vi "HighThroughputReactorCode.vi"() -> ()   [LabVIEW 2021]
uses:
  <vilib>/Utility/error.llb/DialogType.ctl
  839ea58d-a57c-48ce-b4c9-336fce4e4ed7.vi
panel:
  in  "Reactor Selector":T1(ring)
  in  "Stop Program":bool
  in  "Emergency Process Stop":bool
  in  "Reactor Tabs":T2(tab)
  in  "Time Elapsed (s) 1":dbl
  out "Current Cycle 1":string
  out "Completion 1":string
  out "Time Left 1":string="00:00:00"
  in  "Wait Before Start (s) 1":i32
  out "Pressure\nLimit\nTripped 1":bool
  out "Pressure\nTolerance\nTripped 1":bool
  in  "ALD Sequence for Reactor 1":string[][](table)=[["", "", "", ""], ["", "", "", ""], ["", "", "", ""], ["", "", "", ""], ["", "", "", ""], ["", "", "", ""], ["", "", "", ""]]
  in  "Stop / Start Reactor 1":bool
  out "System Idle 1":bool caption="System Idle"
  out "Logging Data 1":bool=TRUE
  in  "ALD Data and Controls":T3(tab)
  out "Pressure Graph 1":dbl(graph) caption="Pressure (mTorr)"
  out "Temperature Graph 1":dbl(graph) caption="Temperature"
  out "Error Trip Time":string
  out "Error Trip Cycle 1":i32
  out "Last Temperature\nRead Success Time":string
  in  "Temp Setpoint":dbl
  in  "Set Temperature":bool=TRUE
  out "Last Cycle Temp\nRead Success":i32
  out "Recorded Pressure":dbl
  out "Table Position Reactor 1":i32
  out "Current Cycle Reactor 1":i32
  out "Queue Reactor 1":refnum<queue>
  out "Timer Reactor 1":i32
  out "Start Time 1":dbl
  out "Save File JSON Connection 1":refnum<file>
  out "Local Connection JSON 1":refnum<file>
  out "Header Connection txt 1":refnum<file>
  out "Save File Connection 1":refnum<file>
  out "Local Connection txt 1":refnum<file>
  in  "GUID 1":string
  in  "Pressure Scale 1":dbl
  in  "Pressure Voltage Correct 1":dbl=5.0
  in  "Load Table Reactor 1":bool
  in  "Save Table Reactor 1":bool
  out "Reactor 1 Errors":errorcluster
  out "Countdown 1":dbl
  in  "Experimental Details 1":string
  in  "Username 1":string
  in  "Time Elapsed (s) 2":dbl
  in  "ALD Data and Controls 2":T3(tab)
  out "Pressure Graph 2":dbl(graph) caption="Pressure (mTorr)"
  out "Temperature Graph 2":dbl(graph) caption="Temperature"
  out "Error Trip Time 2":string
  out "Error Trip Cycle 2":i32
  out "Last Temperature\nRead Success Time 2":string
  in  "Temp Setpoint 2":dbl
  in  "Set Temperature 2":bool=TRUE
  out "Last Cycle Temp\nRead Success 2":i32
  out "Recorded Pressure 2":dbl
  out "Table Position Reactor 2":i32
  out "Current Cycle Reactor 2":i32
  out "Timer Reactor 2":i32
  out "Start Time 2":dbl
  in  "GUID 2":string
  out "Queue Reactor 2":refnum<queue>
  out "Save File JSON Connection 2":refnum<file>
  out "Local Connection JSON 2":refnum<file>
  out "Header Connection txt 2":refnum<file>
  out "Save File Connection 2":refnum<file>
  out "Local Connection txt 2":refnum<file>
  in  "Pressure Scale 2":dbl
  in  "Pressure Voltage Correct 2":dbl=5.0
  out "Reactor 2 Errors":errorcluster
  out "System Idle 2":bool caption="System Idle"
  out "Logging Data 2":bool=TRUE
  out "Pressure\nLimit\nTripped 2":bool
  out "Pressure\nTolerance\nTripped 2":bool
  out "Current Cycle 2":string
  out "Completion 2":string
  out "Time Left 2":string="00:00:00"
  in  "Wait Before Start (s) 2":i32
  in  "ALD Sequence for Reactor 2":string[][](table)=[["", "", "", ""], ["", "", "", ""], ["", "", "", ""], ["", "", "", ""], ["", "", "", ""], ["", "", "", ""], ["", "", "", ""]]
  in  "Stop / Start Reactor 2":bool
  in  "Save Table Reactor 2":bool
  in  "Load Table Reactor 2":bool
  out "Countdown 2":dbl
  in  "Experimental Details 2":string
  in  "Username 2":string
  in  "Time Elapsed (s) 3":dbl
  in  "ALD Data and Controls 3":T3(tab)
  out "Pressure Graph 3":dbl(graph) caption="Pressure (mTorr)"
  out "Temperature Graph 3":dbl(graph) caption="Temperature"
  out "Error Trip Time 3":string
  out "Error Trip Cycle 3":i32
  out "Last Temperature\nRead Success Time 3":string
  in  "Temp Setpoint 3":dbl
  in  "Set Temperature 3":bool=TRUE
  out "Last Cycle Temp\nRead Success 3":i32
  out "Recorded Pressure 3":dbl
  out "Table Position Reactor 3":i32
  out "Current Cycle Reactor 3":i32
  out "Queue Reactor 3":refnum<queue>
  out "Timer Reactor 3":i32
  out "Start Time 3":dbl
  in  "GUID 3":string
  out "Save File JSON Connection 3":refnum<file>
  out "Local Connection JSON 3":refnum<file>
  out "Header Connection txt 3":refnum<file>
  out "Save File Connection 3":refnum<file>
  out "Local Connection txt 3":refnum<file>
  in  "Pressure Scale 3":dbl
  in  "Pressure Voltage Correct 3":dbl=5.0
  out "Reactor 3 Errors":errorcluster
  out "System Idle 3":bool caption="System Idle"
  out "Logging Data 3":bool=TRUE
  out "Pressure\nLimit\nTripped 3":bool
  out "Pressure\nTolerance\nTripped 3":bool
  out "Current Cycle 3":string
  out "Completion 3":string
  out "Time Left 3":string="00:00:00"
  in  "Wait Before Start (s) 3":i32
  in  "ALD Sequence for Reactor 3":string[][](table)=[["", "", "", ""], ["", "", "", ""], ["", "", "", ""], ["", "", "", ""], ["", "", "", ""], ["", "", "", ""], ["", "", "", ""]]
  in  "Stop / Start Reactor 3":bool
  in  "Load Table Reactor 3":bool
  out "Countdown 3":dbl
  in  "Experimental Details 3":string
  in  "Username 3":string
  in  "Save Table Reactor 3":bool
  in  "Time Elapsed (s) 4":dbl
  in  "ALD Data and Controls 4":T3(tab)
  out "Pressure Graph 4":dbl(graph) caption="Pressure (mTorr)"
  out "Temperature Graph 4":dbl(graph) caption="Temperature"
  out "Error Trip Time 4":string
  out "Error Trip Cycle 4":i32
  out "Last Temperature\nRead Success Time 4":string
  in  "Temp Setpoint 4":dbl
  in  "Set Temperature 4":bool=TRUE
  out "Last Cycle Temp\nRead Success 4":i32
  out "Recorded Pressure 4":dbl
  out "Table Position Reactor 4":i32
  out "Current Cycle Reactor 4":i32
  out "Timer Reactor 4":i32
  out "Start Time 4":dbl
  in  "GUID 4":string
  out "Queue Reactor 4":refnum<queue>
  out "Save File JSON Connection 4":refnum<file>
  out "Local Connection JSON 4":refnum<file>
  out "Header Connection txt 4":refnum<file>
  out "Save File Connection 4":refnum<file>
  out "Local Connection txt 4":refnum<file>
  in  "Pressure Scale 4":dbl
  in  "Pressure Voltage Correct 4":dbl=5.0
  out "Reactor 4 Errors":errorcluster
  out "System Idle 4":bool caption="System Idle"
  out "Logging Data 4":bool=TRUE
  out "Pressure\nLimit\nTripped 4":bool
  out "Pressure\nTolerance\nTripped 4":bool
  out "Current Cycle 4":string
  out "Completion 4":string
  out "Time Left 4":string="00:00:00"
  in  "Wait Before Start (s) 4":i32
  in  "ALD Sequence for Reactor 4":string[][](table)=[["", "", "", ""], ["", "", "", ""], ["", "", "", ""], ["", "", "", ""], ["", "", "", ""], ["", "", "", ""], ["", "", "", ""]]
  in  "Stop / Start Reactor 4":bool
  out "Countdown 4":dbl
  in  "Experimental Details 4":string
  in  "Username 4":string
  in  "Load Table Reactor 4":bool
  in  "Save Table Reactor 4":bool
  in  "Time Elapsed (s) 5":dbl
  in  "ALD Data and Controls 5":T3(tab)
  out "Pressure Graph 5":dbl(graph) caption="Pressure (mTorr)"
  out "Temperature Graph 5":dbl(graph) caption="Temperature"
  out "Error Trip Time 5":string
  out "Error Trip Cycle 5":i32
  out "Last Temperature\nRead Success Time 5":string
  in  "Temp Setpoint 5":dbl
  in  "Set Temperature 5":bool=TRUE
  out "Last Cycle Temp\nRead Success 5":i32
  out "Recorded Pressure 5":dbl
  out "Table Position Reactor 5":i32
  out "Current Cycle Reactor 5":i32
  out "Timer Reactor 5":i32
  out "Start Time 5":dbl
  in  "GUID 5":string
  out "Queue Reactor 5":refnum<queue>
  out "Save File JSON Connection 5":refnum<file>
  out "Local Connection JSON 5":refnum<file>
  out "Header Connection txt 5":refnum<file>
  out "Save File Connection 5":refnum<file>
  out "Local Connection txt 5":refnum<file>
  in  "Pressure Scale 5":dbl
  in  "Pressure Voltage Correct 5":dbl=5.0
  out "Reactor 5 Errors":errorcluster
  out "System Idle 5":bool caption="System Idle"
  out "Logging Data 5":bool=TRUE
  out "Pressure\nLimit\nTripped 5":bool
  out "Pressure\nTolerance\nTripped 5":bool
  out "Current Cycle 5":string
  out "Completion 5":string
  out "Time Left 5":string="00:00:00"
  in  "Wait Before Start (s) 5":i32
  in  "ALD Sequence for Reactor 5":string[][](table)=[["", "", "", ""], ["", "", "", ""], ["", "", "", ""], ["", "", "", ""], ["", "", "", ""], ["", "", "", ""], ["", "", "", ""]]
  in  "Stop / Start Reactor 5":bool
  out "Countdown 5":dbl
  in  "Experimental Details 5":string
  in  "Username 5":string
  in  "Load Table Reactor 5":bool
  in  "Save Table Reactor 5":bool
  in  "Time Elapsed (s) 6":dbl
  in  "ALD Data and Controls 6":T3(tab)
  out "Pressure Graph 6":dbl(graph) caption="Pressure (mTorr)"
  out "Temperature Graph 6":dbl(graph) caption="Temperature"
  out "Error Trip Time 6":string
  out "Error Trip Cycle 6":i32
  out "Last Temperature\nRead Success Time 6":string
  in  "Temp Setpoint 6":dbl
  in  "Set Temperature 6":bool=TRUE
  out "Last Cycle Temp\nRead Success 6":i32
  out "Recorded Pressure 6":dbl
  out "Table Position Reactor 6":i32
  out "Current Cycle Reactor 6":i32
  out "Queue Reactor 6":refnum<queue>
  out "Timer Reactor 6":i32
  out "Start Time 6":dbl
  in  "GUID 6":string
  out "Save File JSON Connection 6":refnum<file>
  out "Local Connection JSON 6":refnum<file>
  out "Header Connection txt 6":refnum<file>
  out "Save File Connection 6":refnum<file>
  out "Local Connection txt 6":refnum<file>
  in  "Pressure Scale 6":dbl
  in  "Pressure Voltage Correct 6":dbl=5.0
  out "Reactor 6 Errors":errorcluster
  out "System Idle 6":bool caption="System Idle"
  out "Logging Data 6":bool=TRUE
  out "Pressure\nLimit\nTripped 6":bool
  out "Pressure\nTolerance\nTripped 6":bool
  out "Current Cycle 6":string
  out "Completion 6":string
  out "Time Left 6":string="00:00:00"
  in  "Wait Before Start (s) 6":i32
  in  "ALD Sequence for Reactor 6":string[][](table)=[["", "", "", ""], ["", "", "", ""], ["", "", "", ""], ["", "", "", ""], ["", "", "", ""], ["", "", "", ""], ["", "", "", ""]]
  in  "Stop / Start Reactor 6":bool
  in  "Load Table Reactor 6":bool
  out "Countdown 6":dbl
  in  "Experimental Details 6":string
  in  "Username 6":string
  in  "Save Table Reactor 6":bool
  out "Tempurature Error":errorcluster
  in  "Manual 44":bool
  in  "Manual 43":bool
  in  "Manual 42":bool
  in  "Manual 41":bool
  in  "Manual 40":bool
  in  "Manual 39":bool
  in  "Manual 38":bool
  in  "Manual 37":bool
  in  "Manual 36":bool
  in  "Manual 35":bool
  in  "Manual 34":bool
  in  "Manual 33":bool
  in  "Manual 32":bool
  in  "Manual 31":bool
  in  "Manual 30":bool
  in  "Manual 29":bool
  in  "Manual 28":bool
  in  "Manual 27":bool
  in  "Manual 26":bool
  in  "Manual 25":bool
  in  "Manual 24":bool
  in  "Manual 23":bool
  in  "Manual 22":bool
  in  "Manual 21":bool
  in  "Manual 20":bool
  in  "Manual 19":bool
  in  "Manual 18":bool
  in  "Manual 17":bool
  in  "Manual 16":bool
  in  "Manual 15":bool
  in  "Manual 14":bool
  in  "Manual 13":bool
  out "Chamber 6 Lock Claimed":bool
  out "Chamber 5 Lock Claimed":bool
  out "Chamber 4 Lock Claimed":bool
  out "Chamber 3 Lock Claimed":bool
  in  "Manual Override Chamber 6":bool
  in  "Manual Override Chamber 5":bool
  in  "Manual Override Chamber 4":bool
  in  "Manual Override Chamber 3":bool
  in  "Manual Override\nShared2":bool
  in  "Manual Override\nShared1":bool
  in  "Manual Override\nPumps":bool
  out "Chamber 2 Lock Claimed":bool
  in  "Manual 7":bool
  in  "Manual 12":bool
  in  "Manual 11":bool
  in  "Manual 10":bool
  in  "Manual 9":bool
  in  "Manual Override Chamber 2":bool
  in  "Manual 8":bool
  in  "Manual 1":bool
  in  "Manual 6":bool
  out "Shared 2\nLock Claimed":bool
  out "Shared 1\nLock Claimed":bool
  in  "Manual 5":bool
  in  "Manual 4":bool
  in  "Manual 3":bool
  out "Chamber 1 Lock Claimed":bool
  in  "Manual Override Chamber 1":bool
  out "Pump\nLock Claimed":bool
  in  "Manual 2":bool
  out "Pressure (mTorr) 1":dbl
  out "Pressure (mTorr) 2":dbl
  out "Pressure (mTorr) 3":dbl
  out "Pressure (mTorr) 4":dbl
  out "Pressure (mTorr) 5":dbl
  out "Pressure (mTorr) 6":dbl
  out "Current Valve State":bool[](array[boolean])
  in  "Manual 45":bool
  in  "Manual 46":bool
  in  "Manual 47":bool
  in  "Manual 48":bool
  out "Valve 45":bool
  out "Valve 46":bool
  out "Valve 47":bool
  out "Valve 48":bool
  out "Running Reactor 6":bool
  out "Running Reactor 5":bool
  out "Running Reactor 4":bool
  out "Running Reactor 3":bool
  out "Running Reactor 2":bool
  out "Running Reactor 1":bool
  out "Valve 44":bool
  out "Valve 43":bool
  out "Valve 42":bool
  out "Valve 41":bool
  out "Valve 40":bool
  out "Valve 39":bool
  out "Valve 38":bool
  out "Valve 37":bool
  out "Valve 36":bool
  out "Valve 35":bool
  out "Valve 34":bool
  out "Valve 33":bool
  out "Valve 32":bool
  out "Valve 31":bool
  out "Valve 30":bool
  out "Valve 29":bool
  out "Valve 28":bool
  out "Valve 27":bool
  out "Valve 26":bool
  out "Valve 25":bool
  out "Valve 24":bool
  out "Valve 23":bool
  out "Valve 22":bool
  out "Valve 21":bool
  out "Valve 20":bool
  out "Valve 19":bool
  out "Valve 18":bool
  out "Valve 17":bool
  out "Valve 16":bool
  out "Valve 15":bool
  out "Valve 14":bool
  out "Valve 13":bool
  out "Valve 12":bool
  out "Valve 11":bool
  out "Valve 10":bool
  out "Valve 9":bool
  out "Valve 8":bool
  out "Valve 7":bool
  out "Valve 6":bool
  out "Valve 5":bool
  out "Valve 4":bool
  out "Valve 3":bool
  out "Valve 1":bool
  out "Valve 2":bool
  out "System Log":string[](array[string])
  in  "Debug Mode":bool
  in  "Valve Close Delay":i32=1000
  out "Pressure Tolerance Tripped Array":refnum<vi>[](array[refnum])
  out "Pressure Limit Tripped Array":refnum<vi>[](array[refnum])
  out "Current Cycle Display Array":refnum<vi>[](array[refnum])
  out "Completion Array":refnum<vi>[](array[refnum])
  out "Time Left Array":refnum<vi>[](array[refnum])
  out "Wait Before Start Array":refnum<vi>[](array[refnum])
  out "ALD Sequence for Reactor Array":refnum<vi>[](array[refnum])
  out "Start Stop Reactor Array":refnum<vi>[](array[refnum])
  out "Table Position Reactor Array":refnum<vi>[](array[refnum])
  out "Current Cycle Reactor Array":refnum<vi>[](array[refnum])
  out "System Idle Array":refnum<vi>[](array[refnum])
  out "Logging Data Array":refnum<vi>[](array[refnum])
  out "Reactor Errors Array":refnum<vi>[](array[refnum])
  out "Pressure Graph Array":refnum<vi>[](array[refnum])
  out "Temperature Graph Array":refnum<vi>[](array[refnum])
  out "Recorded Pressure Array":refnum<vi>[](array[refnum])
  out "Last Cycle Temp Read Success Array":refnum<vi>[](array[refnum])
  in  "Lock Reentrance Rate":i32=100
  out "Pump Shared Lock\nClaimed Array":refnum<vi>[](array[refnum])
  out "Number of Reactors":i32=6
  out "Valves Per Reactor":i32=6
  in  "Plot Temp":bool
  in  "Pressure Tolerance":dbl=400.0
  in  "Pressure Limit":dbl=25000.0
  out "Experimental Details Array":refnum<vi>[](array[refnum])
  out "Username Array":refnum<vi>[](array[refnum])
  out "Save File Connection Array":refnum<vi>[](array[refnum])
  out "Valves on Shared 1":i32=4
  out "Valves on Shared 2":i32=4
  out "Pump Valves":i32[](array[numeric])
  out "N2 Valves":i32[](array[numeric])
  in  "Default Purge":bool=TRUE
  out "Save Table Reactor Array":refnum<vi>[](array[refnum])
  out "Load Table Reactor Array":refnum<vi>[](array[refnum])
  out "Pressure (mTorr) Array":refnum<vi>[](array[refnum])
  out "Save File JSON Connection Array":refnum<vi>[](array[refnum])
  out "Valves on Shared Lines":i32=4
  out "Number of Shared Lines":i32=2
  out "Shared Manual Valve Array":refnum<vi>[](array[refnum])
  out "Timer Reactor Array":refnum<vi>[](array[refnum])
  out "Local Connection txt Array":refnum<vi>[](array[refnum])
  out "Queue Array":refnum<vi>[](array[refnum])
  out "Header Connection txt Array":refnum<vi>[](array[refnum])
  out "Time Elapsed Array":refnum<vi>[](array[refnum])
  out "Local Connection JSON Array":refnum<vi>[](array[refnum])
  out "GUID array":refnum<vi>[](array[refnum])
  out "Queue JSON Object":refnum<queue>
  out "Save JSON log Connection":refnum<file>
  out "date on current file":string
  out "Current Locks":i32[](array[numeric])
  out "Chamber Lock Claimed Array":refnum<vi>[](array[refnum])
  out "Last Temperature\nReat Success Time\nArray":refnum<vi>[](array[refnum])
  out "Manual Override\nPump Shared Array":refnum<vi>[](array[refnum])
  out "Error Trip Cycle\nArray":refnum<vi>[](array[refnum])
  out "Countdown Array":refnum<vi>[](array[refnum])
  out "Error Trip Time\nArray":refnum<vi>[](array[refnum])
  out "Temp Setpoint Array":refnum<vi>[](array[refnum])
  out "Set Temperature Array":refnum<vi>[](array[refnum])
  out "Manual Override\nChamber Array":refnum<vi>[](array[refnum])
  out "Queue System":refnum<queue>
  out "Maximum Possible\nReactors":i32
  out "Pressure Scale Array":refnum<vi>[](array[refnum])
  out "Pressure Voltage\nCorrect Array":refnum<vi>[](array[refnum])
  out "Maximum Possible\nShared Lines":i32
  out "Running Reactor\nIndicator Array":refnum<vi>[](array[refnum])
  out "Valve Indicator Array":refnum<vi>[](array[refnum])
  out "Maximum Possible\nValves Per Shared Line":i32
  out "Maximum Possible\nValves Per Reactor":i32
  out "Reactor Name":string
  out "System Constants":T4
  out "Manual Valve Array":refnum<vi>[](array[refnum])
  out "Start Time Array":refnum<vi>[](array[refnum])
  # "Valve Designations"
  # "Don't use\n1: Pump\n2: N2"
  # "52: Shared DEZ\n53: Shared TMA\n54: Shared DEDMS"
  # "62: Shared Water\n63: Shared Diol\n64: Ethylene Glycol"
  # "5: <Local Valve 5 Reactant>\n6: <Local Valve 6 Reactant>"
  # "99: Set Temperature\n     (pulse = temp, purge = wait time)"
  # "Reactor 1"
  # "Reactor 3"
  # "Reactor 5"
  # "Reactor 2"
  # "Reactor 4"
  # "Reactor 6"
  # "Shared 2"
  # "Shared 1"
  # "Most Recent"
  # "Least Recent"
  # "Variables"
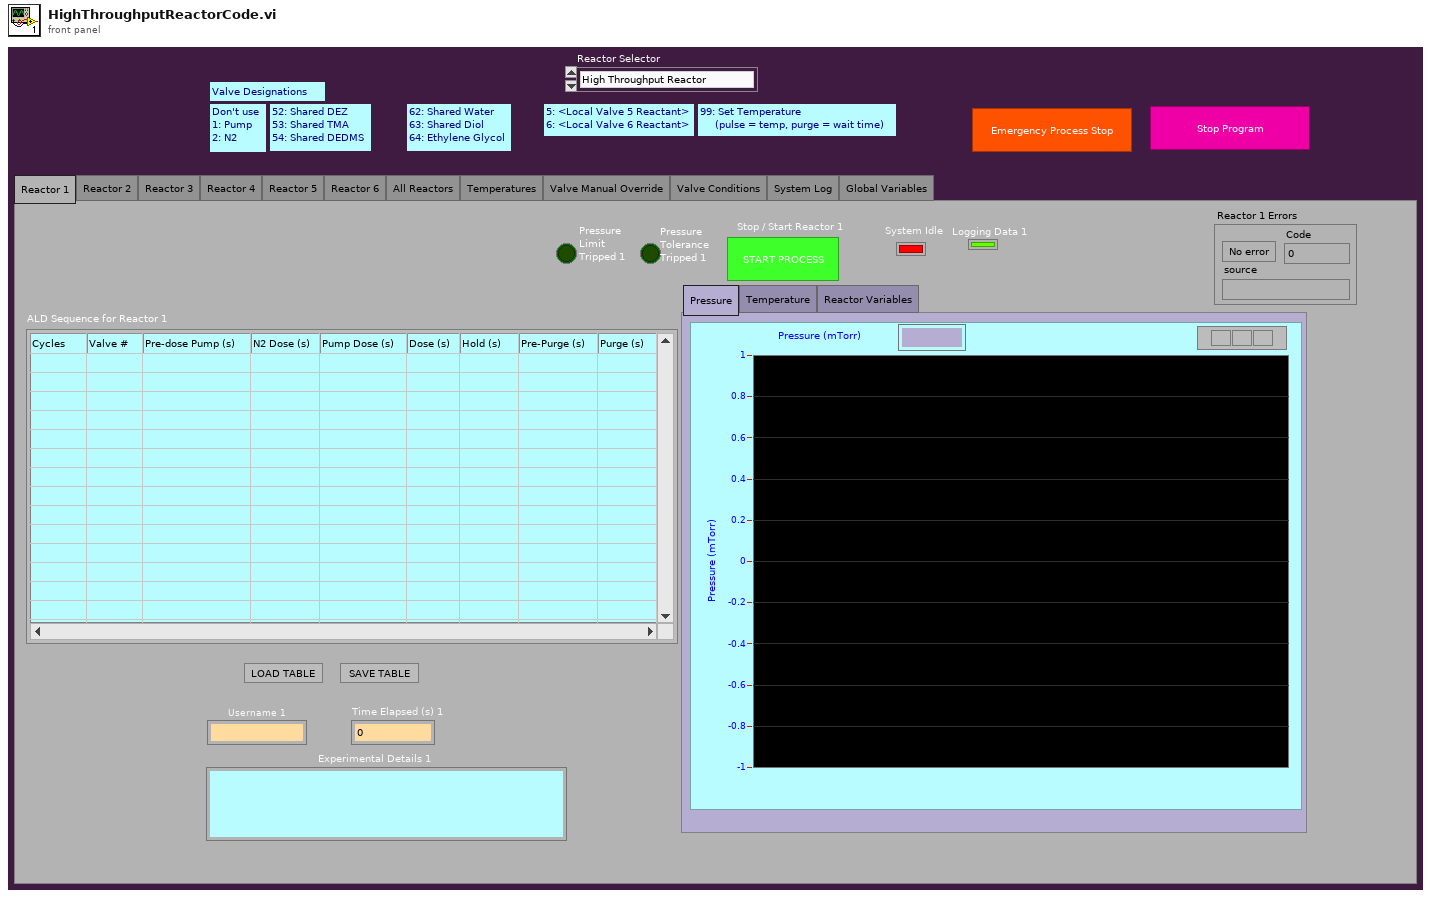
[diagram p1: front panel]
types:
  T1 = enum16{"High Throughput Reactor", "In Situ Reactor", "MLD Reactor"}
  T2 = enum32{"Reactor 1", "Reactor 2", "Reactor 3", "Reactor 4", "Reactor 5", "Reactor 6", "All Reactors", "Temperatures", "Valve Manual Override", "Valve Conditions", "System Log", "Global Variables"}
  T3 = enum32{"Pressure", "Temperature", "Reactor Variables"}
  T4 = cluster{"Valves Per Shared Line":i32, "Number of Reactors":i32, "Valves Per Reactor":i32, "Number of Shared Lines":i32, "Reactor Name":string, "N2 Valves":i32[], "Pump Valves":i32[]}
  T5 = typedef "DialogType.ctl" = u16
  T6 = cluster{"ALD Sequence for Reactor 6":refnum<vi>, "Username 6":refnum<vi>, "Experimental Details 6":refnum<vi>}
  T7 = cluster{"type":string, "meta":string, "payload":cluster{"GUID":string, "valveSequence":i32[][]}}
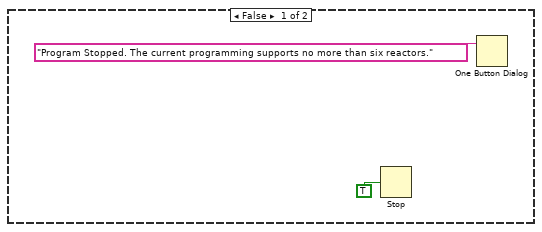
[diagram p2: hidden frame]
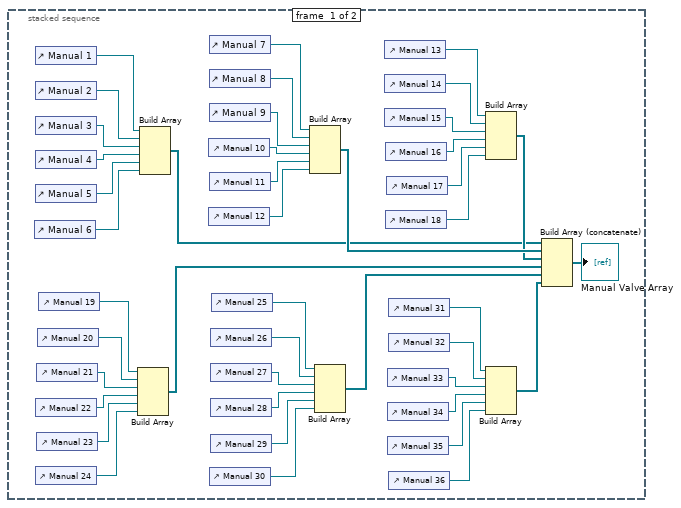
[diagram p3: hidden frame]
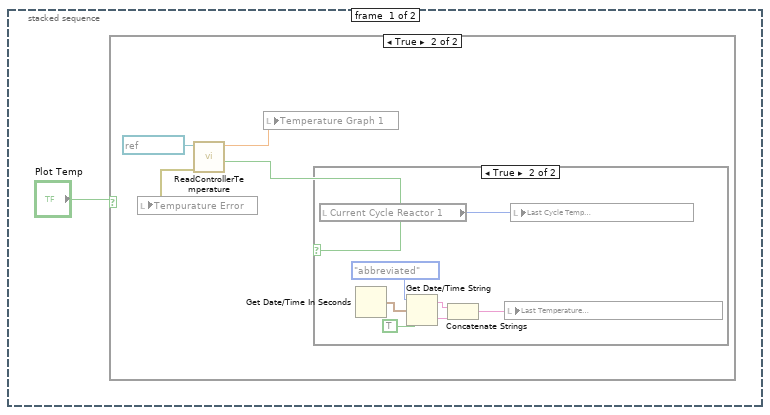
[diagram p11: hidden frame]
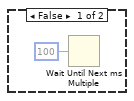
[diagram p12: hidden frame]
diagram:
  w2 = 0.0
  w107 = refnum<file> refnum ("Header Connection txt 1")
  w105 = refnum<file> refnum ("Save File Connection 6")
  w169 = 0
  w81 = ""
  w185 = errorcluster {"status"=FALSE, "code"=0, "source"=""} ("error constant")
  w186 = FALSE
  w187 = FALSE
  w188 = refnum<file> refnum ("Save File Connection 6")
  w189 = ""
  w190 = ""
  w191 = ""
  w192 = 0
  w193 = 0
  w194 = FALSE
  w195 = TRUE
  w196 = FALSE
  # "Temperature Read/Set"
  n1 = flat-sequence {
    tunnel: [w421] -> w80
    tunnel: [w430] -> w65
    tunnel: [w429] -> w64
    tunnel: [w423] -> w63
    tunnel: w80 -> [w440]
    tunnel: w65 -> [w441]
    tunnel: w64 -> [w435]
    tunnel: w63 -> [w431]
    frame #0 {
      w429 = 2
      w430 = 6
      n2 = call "ReactorInitialization.vi"("Reactor Selector"="Reactor Selector") -> ("System Constants"=w418:T4)
      "System Constants" <- w418
      n3 = Unbundle By Name(w418) -> ("Valves Per Shared Line"=→"Valves on Shared 1" →"Valves on Shared 2" →"Valves on Shared Lines":i32, "Number of Reactors"=w421:i32, "Valves Per Reactor"=→"Valves Per Reactor":i32, "Number of Shared Lines"=w423:i32, "Reactor Name"=→"Reactor Name":string, "N2 Valves"=→"N2 Valves":i32[], "Pump Valves"=→"Pump Valves":i32[])
      "Number of Reactors" <- w421
      "Number of Shared Lines" <- w423
      "Maximum Possible\nReactors" <- w430
      "Maximum Possible\nShared Lines" <- w429
      "Maximum Possible\nValves Per Reactor" <- 6 ("Maximum Possible\nValves Per Reactor")
      "Maximum Possible\nValves Per Shared Line" <- 6 ("Maximum Possible\nValves Per Reactor")
    }
    frame #1 {
      # "Initialize Variables"
      n4 = Less Or Equal?(x=w440, y=w441) -> (x <= y?=w438:bool)
      n5 = Greater Than 0?(x=w440) -> (x > 0?=w439:bool)
      n6 = Less Or Equal?(x=w431, y=w435) -> (x <= y?=w437:bool)
      n7 = Greater Or Equal To 0?(x=w431) -> (x >= 0?=w436:bool)
      n8 = And(x=w439, y=w438) -> (x .and. y?=w433:bool)
      n9 = And(x=w436, y=w437) -> (x .and. y?=w434:bool)
      n10 = And(x=w433, y=w434) -> (x .and. y?=w432:bool)
      n11 = case shown="True" w432 {
        tunnel: w440 -> [_ w515]
        tunnel: w431 -> [_ w518]
        frame False {
          n12 = Stop(stop? (T)=TRUE) -> ()
          n13 = One Button Dialog(message="Program Stopped. The current programming supports no more than six reactors.") -> ()  [unwired: 1 in, 1 out]
        }
        frame True {
          # "Remove Unused Buttons from array to be consistent\nwith locks."
          # "Remove Unused Buttons from array to be consistent\nwith locks."
          # "Lock Indicies:\n0 Pump\n1 - S Shared Lines\nS+1 - S+N Reactors"
          # "Disable Reactor Tabs not in use"
          n14 = property on="Reactor Tabs" class="TabCtl (strict)"() -> ("Pages"=w519:refnum<vi>[])  [unwired: 2 in, 2 out]
          n15 = local read "Maximum Possible\nReactors"() -> (w521:i32)
          n16 = stacked-sequence {
            frame #0 {
              n17 = control-ref of="Manual 6"() -> (w535:refnum<vi>)
              n18 = control-ref of="Manual 1"() -> (w528:refnum<vi>)
              n19 = control-ref of="Manual 2"() -> (w529:refnum<vi>)
              n20 = control-ref of="Manual 3"() -> (w532:refnum<vi>)
              n21 = control-ref of="Manual 4"() -> (w533:refnum<vi>)
              n22 = control-ref of="Manual 5"() -> (w534:refnum<vi>)
              n23 = control-ref of="Manual 22"() -> (w552:refnum<vi>)
              n24 = control-ref of="Manual 24"() -> (w554:refnum<vi>)
              n25 = control-ref of="Manual 21"() -> (w551:refnum<vi>)
              n26 = control-ref of="Manual 23"() -> (w553:refnum<vi>)
              n27 = control-ref of="Manual 20"() -> (w550:refnum<vi>)
              n28 = control-ref of="Manual 19"() -> (w549:refnum<vi>)
              n29 = Build Array(w549, w550, w551, w552, w553, w554) -> (w555:refnum<vi>[])
              n30 = Build Array(w528, w529, w532, w533, w534, w535) -> (w531:refnum<vi>[])
              n31 = control-ref of="Manual 10"() -> (w538:refnum<vi>)
              n32 = control-ref of="Manual 12"() -> (w540:refnum<vi>)
              n33 = control-ref of="Manual 7"() -> (w530:refnum<vi>)
              n34 = control-ref of="Manual 8"() -> (w536:refnum<vi>)
              n35 = control-ref of="Manual 9"() -> (w537:refnum<vi>)
              n36 = control-ref of="Manual 11"() -> (w539:refnum<vi>)
              n37 = control-ref of="Manual 30"() -> (w561:refnum<vi>)
              n38 = control-ref of="Manual 26"() -> (w557:refnum<vi>)
              n39 = control-ref of="Manual 27"() -> (w558:refnum<vi>)
              n40 = control-ref of="Manual 28"() -> (w559:refnum<vi>)
              n41 = control-ref of="Manual 29"() -> (w560:refnum<vi>)
              n42 = control-ref of="Manual 25"() -> (w556:refnum<vi>)
              n43 = Build Array(w530, w536, w537, w538, w539, w540) -> (w548:refnum<vi>[])
              n44 = Build Array(w556, w557, w558, w559, w560, w561) -> (w562:refnum<vi>[])
              n45 = control-ref of="Manual 13"() -> (w541:refnum<vi>)
              n46 = control-ref of="Manual 14"() -> (w542:refnum<vi>)
              n47 = control-ref of="Manual 15"() -> (w543:refnum<vi>)
              n48 = control-ref of="Manual 16"() -> (w544:refnum<vi>)
              n49 = control-ref of="Manual 18"() -> (w546:refnum<vi>)
              n50 = control-ref of="Manual 17"() -> (w545:refnum<vi>)
              n51 = control-ref of="Manual 33"() -> (w565:refnum<vi>)
              n52 = control-ref of="Manual 34"() -> (w566:refnum<vi>)
              n53 = control-ref of="Manual 35"() -> (w567:refnum<vi>)
              n54 = control-ref of="Manual 31"() -> (w563:refnum<vi>)
              n55 = control-ref of="Manual 32"() -> (w564:refnum<vi>)
              n56 = control-ref of="Manual 36"() -> (w568:refnum<vi>)
              n57 = Build Array(w541, w542, w543, w544, w545, w546) -> (w547:refnum<vi>[])
              n58 = Build Array(w563, w564, w565, w566, w567, w568) -> (w569:refnum<vi>[])
              n59 = Build Array (concatenate)(w531, w548, w547, w555, w562, w569) -> (→"Manual Valve Array":refnum<vi>[])
            }
            frame #1 {
              n60 = control-ref of="Manual Valve Array"() -> (w571:refnum<vi>)
              n61 = local read "Number of Reactors"() -> (w573:i32)
              n62 = local read "Valves Per Reactor"() -> (w572:i32)
              n63 = property class="Arr (strict)"(reference=w571) -> ("Value"=w570:refnum<vi>[])  [unwired: 1 in, 2 out]
              n64 = Multiply(x=w573, y=w572) -> (x*y=w576:i32)
              n65 = Split 1D Array(array=w570, index=w576) -> (first subarray=w575:refnum<vi>[], second subarray=w574:refnum<vi>[])
              n66 = for {
                tunnel: w575 -> [w580] mode=indexing
                n67 = property class="Bool (strict)"(reference=w580, "Visible"=TRUE) -> ()  [unwired: 1 in, 2 out]
              }
              n68 = for {
                tunnel: w574 -> [w578] mode=indexing
                n69 = property class="Bool (strict)"(reference=w578, "Visible"=FALSE) -> ()  [unwired: 1 in, 2 out]
              }
            }
          }
          n70 = local read "Maximum Possible\nValves Per Reactor"() -> (w509:i32)
          n71 = local read "Maximum Possible\nReactors"() -> (w510:i32)
          n72 = control-ref of="Valve Indicator Array"() -> (w516:refnum<vi>)
          n73 = for {
            tunnel: w519 -> [w623] mode=indexing
            tunnel: w518 -> [w618]
            tunnel: w515 -> [w617]
            n74 = property class="Page"(reference=w623) -> (reference out=w619:refnum<vi>, "TabCaption"=w622:string)  [unwired: 1 in, 1 out]
            n75 = Equal?(x=w622, y="Valve Conditions") -> (x = y?=w620:bool)
            n76 = case shown="True" w620 {
              tunnel: w619 -> [_ w640]
              tunnel: w618 -> [_ w636]
              tunnel: w617 -> [_ w629]
              frame False {
              }
              frame True {
                # "Banner Title\nand Box"
                n77 = property class="Page"(reference=w640) -> ("DecosOnPage"=w639:refnum<vi>[])  [unwired: 1 in, 2 out]
                n78 = Multiply(x=w636, y=2) -> (x*y=w633:i32)
                n79 = Multiply(x=w629, y=2) -> (x*y=w624:i32)
                n80 = Split 1D Array(array=w639, index=4) -> (first subarray=w631:refnum<vi>[], second subarray=w626:refnum<vi>[])
                n81 = Array Subset(array=w631, index=0, length=w633) -> (w634:refnum<vi>[])
                n82 = Array Subset(array=w626, index=0, length=w624) -> (w627:refnum<vi>[])
                n83 = Array Subset(array=w631, index=w633) -> (w632:refnum<vi>[])  [unwired: 1 in]
                n84 = Array Subset(array=w626, index=w624) -> (w628:refnum<vi>[])  [unwired: 1 in]
                n85 = for {
                  tunnel: w634 -> [w648] mode=indexing
                  n86 = property class="Decor"(reference=w648, "Visible"=TRUE) -> ()  [unwired: 1 in, 2 out]
                }
                n87 = for {
                  tunnel: w627 -> [w644] mode=indexing
                  n88 = property class="Decor"(reference=w644, "Visible"=TRUE) -> ()  [unwired: 1 in, 2 out]
                }
                n89 = for {
                  tunnel: w632 -> [w646] mode=indexing
                  n90 = property class="Decor"(reference=w646, "Visible"=FALSE) -> ()  [unwired: 1 in, 2 out]
                }
                n91 = for {
                  tunnel: w628 -> [w642] mode=indexing
                  n92 = property class="Decor"(reference=w642, "Visible"=FALSE) -> ()  [unwired: 1 in, 2 out]
                }
              }
            }
          }
          n93 = control-ref of="Running Reactor\nIndicator Array"() -> (w517:refnum<vi>)
          n94 = local read "Number of Shared Lines"() -> (w500:i32)
          n95 = local read "Valves on Shared Lines"() -> (w501:i32)
          n96 = local read "Number of Reactors"() -> (w507:i32)
          n97 = local read "Valves Per Reactor"() -> (w506:i32)
          n98 = control-ref of="Shared Manual Valve Array"() -> (w494:refnum<vi>)
          n99 = control-ref of="Pump Shared Lock\nClaimed Array"() -> (w470:refnum<vi>)
          n100 = control-ref of="Manual Override\nPump Shared Array"() -> (w469:refnum<vi>)
          n101 = local read "Number of Shared Lines"() -> (w493:i32)
          n102 = local read "Valves on Shared Lines"() -> (w492:i32)
          n103 = control-ref of="Chamber Lock Claimed Array"() -> (w475:refnum<vi>)
          n104 = property class="Arr (strict)"(reference=w516) -> ("Value"=w511:refnum<vi>[])  [unwired: 1 in, 2 out]
          n105 = control-ref of="Manual Override\nChamber Array"() -> (w480:refnum<vi>)
          n106 = control-ref of="Pressure (mTorr) Array"() -> (w489:refnum<vi>)
          n107 = property class="Arr (strict)"(reference=w517) -> ("Value"=w512:refnum<vi>[])  [unwired: 1 in, 2 out]
          n108 = local read "Number of Shared Lines"() -> (w466:i32)
          n109 = property on="Reactor Tabs" class="TabCtl (strict)"() -> ("Pages"=w520:refnum<vi>[])  [unwired: 2 in, 2 out]
          n110 = property class="Arr (strict)"(reference=w475) -> ("Value"=w476:refnum<vi>[])  [unwired: 1 in, 2 out]
          n111 = property class="Arr (strict)"(reference=w469) -> (reference out=w446:refnum<vi>, "Value"=w471:refnum<vi>[])  [unwired: 1 in, 1 out]
          n112 = local read "Number of Reactors"() -> (w477:i32)
          n113 = property class="Arr (strict)"(reference=w470) -> (reference out=w448:refnum<vi>, "Value"=w474:refnum<vi>[])  [unwired: 1 in, 1 out]
          n114 = property class="Arr (strict)"(reference=w489) -> ("Value"=w485:refnum<vi>[])  [unwired: 1 in, 2 out]
          n115 = property class="Arr (strict)"(reference=w480) -> ("Value"=w484:refnum<vi>[])  [unwired: 1 in, 2 out]
          n116 = local read "Number of Reactors"() -> (w486:i32)
          n117 = local read "Number of Reactors"() -> (w483:i32)
          n118 = Subtract(x=w521, y=w515) -> (x-y=w523:i32)
          n119 = Multiply(x=w510, y=w509) -> (x*y=w508:i32)
          n120 = Multiply(x=w507, y=w506) -> (x*y=w502:i32)
          n121 = Multiply(x=w500, y=w501) -> (x*y=w496:i32)
          n122 = Multiply(x=w493, y=w492) -> (x*y=w491:i32)
          n123 = property class="Arr (strict)"(reference=w494) -> (reference out=w444:refnum<vi>, "Value"=w495:refnum<vi>[])  [unwired: 1 in, 1 out]
          n124 = Split 1D Array(array=w511, index=w508) -> (first subarray=w503:refnum<vi>[], second subarray=w497:refnum<vi>[])
          n125 = Split 1D Array(array=w512, index=w515) -> (first subarray=w514:refnum<vi>[], second subarray=w513:refnum<vi>[])
          n126 = local read "Number of Shared Lines"() -> (w464:i32)
          n127 = Array Subset(array=w520, index=w515, length=w523) -> (w524:refnum<vi>[])
          n128 = Array Subset(array=w520, index=0, length=w515) -> (w525:refnum<vi>[])
          n129 = Array Subset(array=w520, index=w521) -> (w522:refnum<vi>[])  [unwired: 1 in]
          n130 = local read "Number of Reactors"() -> (w455:i32)
          n131 = local read "Number of Shared Lines"() -> (w461:i32)
          n132 = Increment(x=w466) -> (x+1=w467:i32)
          n133 = local read "Valves on Shared Lines"() -> (w460:i32)
          n134 = for {
            tunnel: w514 -> [w616] mode=indexing
            n135 = property class="Bool (strict)"(reference=w616, "Visible"=TRUE) -> ()  [unwired: 1 in, 2 out]
          }
          n136 = Increment(x=w466) -> (x+1=w468:i32)
          n137 = local read "Number of Reactors"() -> (w456:i32)
          n138 = local read "Valves Per Reactor"() -> (w459:i32)
          n139 = for {
            tunnel: w525 -> [w652] mode=indexing
            n140 = property class="Page"(reference=w652, "PageVis"=TRUE ("Page Visible")) -> ()  [unwired: 1 in, 2 out]
          }
          n141 = for {
            tunnel: w524 -> [w654] mode=indexing
            n142 = property class="Page"(reference=w654, "PageVis"=FALSE ("Page Visible")) -> ()  [unwired: 1 in, 2 out]
          }
          n143 = for {
            tunnel: w522 -> [w650] mode=indexing
            n144 = property class="Page"(reference=w650, "PageVis"=TRUE ("Page Visible")) -> ()  [unwired: 1 in, 2 out]
          }
          n145 = Split 1D Array(array=w476, index=w477) -> (first subarray=w478:refnum<vi>[], second subarray=w479:refnum<vi>[])
          n146 = Split 1D Array(array=w471, index=w468) -> (first subarray=w447:refnum<vi>[], second subarray=w472:refnum<vi>[])
          n147 = Split 1D Array(array=w474, index=w467) -> (first subarray=w449:refnum<vi>[], second subarray=w473:refnum<vi>[])
          n148 = Split 1D Array(array=w495, index=w491) -> (first subarray=w445:refnum<vi>[], second subarray=w490:refnum<vi>[])
          n149 = Split 1D Array(array=w503, index=w502) -> (first subarray=w504:refnum<vi>[], second subarray=w505:refnum<vi>[])
          n150 = Split 1D Array(array=w497, index=w496) -> (first subarray=w499:refnum<vi>[], second subarray=w498:refnum<vi>[])
          n151 = Split 1D Array(array=w485, index=w486) -> (first subarray=w487:refnum<vi>[], second subarray=w488:refnum<vi>[])
          n152 = Split 1D Array(array=w484, index=w483) -> (first subarray=w482:refnum<vi>[], second subarray=w481:refnum<vi>[])
          n153 = Add(x=1, y=w464) -> (x+y=w465:i32)
          n154 = for {
            tunnel: w504 -> [w612] mode=indexing
            n155 = property class="Bool (strict)"(reference=w612, "Visible"=TRUE) -> ()  [unwired: 1 in, 2 out]
          }
          n156 = for {
            tunnel: w499 -> [w608] mode=indexing
            n157 = property class="Bool (strict)"(reference=w608, "Visible"=TRUE) -> ()  [unwired: 1 in, 2 out]
          }
          n158 = for {
            tunnel: w478 -> [w592] mode=indexing
            n159 = property class="Bool (strict)"(reference=w592, "Visible"=TRUE) -> ()  [unwired: 1 in, 2 out]
          }
          n160 = for {
            tunnel: w447 -> [w584] mode=indexing
            n161 = property class="Bool (strict)"(reference=w584, "Visible"=TRUE) -> ()  [unwired: 1 in, 2 out]
          }
          n162 = for {
            tunnel: w449 -> [w588] mode=indexing
            n163 = property class="Bool (strict)"(reference=w588, "Visible"=TRUE) -> ()  [unwired: 1 in, 2 out]
          }
          n164 = for {
            tunnel: w445 -> [w604] mode=indexing
            n165 = property class="Bool (strict)"(reference=w604, "Visible"=TRUE) -> ()  [unwired: 1 in, 2 out]
          }
          n166 = for {
            tunnel: w487 -> [w600] mode=indexing
            n167 = property class="DigNum (strict)"(reference=w600, "Visible"=TRUE) -> ()  [unwired: 1 in, 2 out]
          }
          n168 = for {
            tunnel: w482 -> [w596] mode=indexing
            n169 = property class="Bool (strict)"(reference=w596, "Visible"=TRUE) -> ()  [unwired: 1 in, 2 out]
          }
          n170 = property class="Arr (strict)"(reference=w444, "Value"=w445) -> ()  [unwired: 1 in, 2 out]
          n171 = property class="Arr (strict)"(reference=w446, "Value"=w447) -> ()  [unwired: 1 in, 2 out]
          n172 = Add(x=w465, y=w455) -> (x+y=w453:i32)
          n173 = property class="Arr (strict)"(reference=w448, "Value"=w449) -> ()  [unwired: 1 in, 2 out]
          n174 = Multiply(x=w456, y=w459) -> (x*y=w458:i32)
          n175 = Multiply(x=w461, y=w460) -> (x*y=w462:i32)
          n176 = Initialize Array(0 ("element"), w453) -> (→"Current Locks":i32[])
          n177 = for {
            tunnel: w513 -> [w614] mode=indexing
            n178 = property class="Bool (strict)"(reference=w614, "Visible"=FALSE) -> ()  [unwired: 1 in, 2 out]
          }
          n179 = Add(x=w458, y=w462) -> (x+y=w463:i32)
          n180 = Initialize Array(FALSE, w463) -> (→"Current Valve State":bool[])
          n181 = for {
            tunnel: w505 -> [w610] mode=indexing
            n182 = property class="Bool (strict)"(reference=w610, "Visible"=FALSE) -> ()  [unwired: 1 in, 2 out]
          }
          n183 = for {
            tunnel: w498 -> [w606] mode=indexing
            n184 = property class="Bool (strict)"(reference=w606, "Visible"=FALSE) -> ()  [unwired: 1 in, 2 out]
          }
          n185 = for {
            tunnel: w490 -> [w602] mode=indexing
            n186 = property class="Bool (strict)"(reference=w602, "Visible"=FALSE) -> ()  [unwired: 1 in, 2 out]
          }
          n187 = for {
            tunnel: w488 -> [w598] mode=indexing
            n188 = property class="DigNum (strict)"(reference=w598, "Visible"=FALSE) -> ()  [unwired: 1 in, 2 out]
          }
          n189 = for {
            tunnel: w479 -> [w590] mode=indexing
            n190 = property class="Bool (strict)"(reference=w590, "Visible"=FALSE) -> ()  [unwired: 1 in, 2 out]
          }
          n191 = for {
            tunnel: w481 -> [w594] mode=indexing
            n192 = property class="Bool (strict)"(reference=w594, "Visible"=FALSE) -> ()  [unwired: 1 in, 2 out]
          }
          n193 = for {
            tunnel: w472 -> [w582] mode=indexing
            n194 = property class="Bool (strict)"(reference=w582, "Visible"=FALSE) -> ()  [unwired: 1 in, 2 out]
          }
          n195 = for {
            tunnel: w473 -> [w586] mode=indexing
            n196 = property class="Bool (strict)"(reference=w586, "Visible"=FALSE) -> ()  [unwired: 1 in, 2 out]
          }
        }
      }
      n197 = control-ref of="Shared Manual Valve Array"() -> ()  [unwired: 1 out]
    }
    frame #2 {
      n198 = Wait (ms)(milliseconds to wait=u32 1000) -> ()  [unwired: 1 out]
    }
    frame #3 {
      w708 = T5 0 items=["no dialog", "OK message", "continue or stop message", "OK message + warnings", "continue/stop + warnings"] ("type of dialog (OK msg:1)")
      w722 = T5 0 items=["no dialog", "OK message", "continue or stop message", "OK message + warnings", "continue/stop + warnings"] ("type of dialog (OK msg:1)")
      w760 = T5 0 items=["no dialog", "OK message", "continue or stop message", "OK message + warnings", "continue/stop + warnings"] ("type of dialog (OK msg:1)")
      w785 = T5 0 items=["no dialog", "OK message", "continue or stop message", "OK message + warnings", "continue/stop + warnings"] ("type of dialog (OK msg:1)")
      w790 = T5 0 items=["no dialog", "OK message", "continue or stop message", "OK message + warnings", "continue/stop + warnings"] ("type of dialog (OK msg:1)")
      w812 = T5 0 items=["no dialog", "OK message", "continue or stop message", "OK message + warnings", "continue/stop + warnings"] ("type of dialog (OK msg:1)")
      w821 = T5 0 items=["no dialog", "OK message", "continue or stop message", "OK message + warnings", "continue/stop + warnings"] ("type of dialog (OK msg:1)")
      w841 = T5 0 items=["no dialog", "OK message", "continue or stop message", "OK message + warnings", "continue/stop + warnings"] ("type of dialog (OK msg:1)")
      w846 = T5 0 items=["no dialog", "OK message", "continue or stop message", "OK message + warnings", "continue/stop + warnings"] ("type of dialog (OK msg:1)")
      w859 = T5 0 items=["no dialog", "OK message", "continue or stop message", "OK message + warnings", "continue/stop + warnings"] ("type of dialog (OK msg:1)")
      w884 = T5 0 items=["no dialog", "OK message", "continue or stop message", "OK message + warnings", "continue/stop + warnings"] ("type of dialog (OK msg:1)")
      w898 = T5 0 items=["no dialog", "OK message", "continue or stop message", "OK message + warnings", "continue/stop + warnings"] ("type of dialog (OK msg:1)")
      w919 = T5 0 items=["no dialog", "OK message", "continue or stop message", "OK message + warnings", "continue/stop + warnings"] ("type of dialog (OK msg:1)")
      w943 = T5 0 items=["no dialog", "OK message", "continue or stop message", "OK message + warnings", "continue/stop + warnings"] ("type of dialog (OK msg:1)")
      w952 = T5 0 items=["no dialog", "OK message", "continue or stop message", "OK message + warnings", "continue/stop + warnings"] ("type of dialog (OK msg:1)")
      w966 = T5 0 items=["no dialog", "OK message", "continue or stop message", "OK message + warnings", "continue/stop + warnings"] ("type of dialog (OK msg:1)")
      # "Manual Override Loop"
      # "Reactor Running Indicator: Constantly updated to the current reactor state"
      # "Valve Indicators - Constantly updated to the current valve state"
      # "Default Process"
      # "Loop to Run a Process"
      # "Loop to Stop a Process"
      # "Loop to Start a Process"
      # "Save System JSON Queue into File"
      # "Manual Override Locks"
      # "Emergency Stop"
      # "Manual Override Button Enable Shared"
      # "Manual Override Button Enable/Disable"
      # "Save System Text Queue into Text Queue"
      # "Loop to Check If Pressure Limit Tripped"
      # "Record Pressure Data Into Queue"
      # "Loop to Consume and Save Pressure Readings"
      # "Loop to Tick the Countdown Timer"
      # "Loop to Load/Save Process Table"
      n199 = control-ref of="Manual Valve Array"() -> (w669:refnum<vi>)
      n200 = control-ref of="Start Time Array"() -> (w657:refnum<vi>)
      n201 = control-ref of="System Idle Array"() -> (w712:refnum<vi>)
      n202 = control-ref of="Recorded Pressure Array"() -> (w744:refnum<vi>)
      n203 = control-ref of="Timer Reactor Array"() -> (w746:refnum<vi>)
      n204 = control-ref of="Chamber Lock Claimed Array"() -> (w989:refnum<vi>)
      n205 = control-ref of="Save File JSON Connection Array"() -> (w946:refnum<vi>)
      n206 = control-ref of="Start Stop Reactor Array"() -> (w713:refnum<vi>)
      n207 = control-ref of="Load Table Reactor Array"() -> (w982:refnum<vi>)
      n208 = local read "Number of Shared Lines"() -> (w685:i32)
      n209 = control-ref of="Current Cycle Reactor Array"() -> (w890:refnum<vi>)
      n210 = local read "Valves on Shared Lines"() -> (w843:i32)
      n211 = local read "Reactor Name"() -> (w677:string)
      n212 = local read "Lock Reentrance Rate"() -> (w710:i32)
      n213 = local read "Valves Per Reactor"() -> (w671:i32)
      n214 = control-ref of="Pressure Scale Array"() -> (w692:refnum<vi>)
      n215 = control-ref of="Pressure Voltage\nCorrect Array"() -> (w693:refnum<vi>)
      n216 = local read "Number of Reactors"() -> (w672:i32)
      n217 = control-ref of="Shared Manual Valve Array"() -> (w844:refnum<vi>)
      n218 = control-ref of="Emergency Process Stop"() -> (w833:refnum<vi>)
      n219 = property class="Arr (strict)"(reference=w712) -> ("Value"=w777:refnum<vi>[])  [unwired: 1 in, 2 out]
      n220 = property class="Arr (strict)"(reference=w989) -> ("Value"=w828:refnum<vi>[])  [unwired: 1 in, 2 out]
      n221 = property class="Arr (strict)"(reference=w744) -> ("Value"=w743:refnum<vi>[])  [unwired: 1 in, 2 out]
      n222 = property class="Arr (strict)"(reference=w746) -> ("Value"=w745:refnum<vi>[])  [unwired: 1 in, 2 out]
      n223 = property class="Arr (strict)"(reference=w946) -> ("Value"=w908:refnum<vi>[])  [unwired: 1 in, 2 out]
      n224 = property class="Arr (strict)"(reference=w713) -> (reference out=w830:refnum<vi>, "Value"=w983:refnum<vi>[])  [unwired: 1 in, 1 out]
      n225 = property class="Arr (strict)"(reference=w657) -> ("Value"=w662:refnum<vi>[])  [unwired: 1 in, 2 out]
      n226 = property class="Arr (strict)"(reference=w669) -> ("Value"=w670:refnum<vi>[])  [unwired: 1 in, 2 out]
      n227 = property class="Arr (strict)"(reference=w890) -> ("Value"=w661:refnum<vi>[])  [unwired: 1 in, 2 out]
      n228 = property class="Arr (strict)"(reference=w982) -> ("Value"=w981:refnum<vi>[])  [unwired: 1 in, 2 out]
      n229 = property class="Arr (strict)"(reference=w844) -> ("Value"=w868:refnum<vi>[])  [unwired: 1 in, 2 out]
      n230 = property class="Arr (strict)"(reference=w693) -> ("Value"=w691:refnum<vi>[])  [unwired: 1 in, 2 out]
      n231 = property class="Arr (strict)"(reference=w692) -> ("Value"=w690:refnum<vi>[])  [unwired: 1 in, 2 out]
      n232 = local read "Reactor Selector"() -> (w673:T1)
      n233 = control-ref of="Logging Data Array"() -> (w944:refnum<vi>)
      n234 = control-ref of="Countdown Array"() -> (w778:refnum<vi>)
      n235 = control-ref of="Valve Close Delay"() -> (w742:refnum<vi>)
      n236 = control-ref of="Wait Before Start Array"() -> (w773:refnum<vi>)
      n237 = control-ref of="Error Trip Time Array"() -> (w887:refnum<vi>)
      n238 = control-ref of="Pump Shared Lock\nClaimed Array"() -> (w832:refnum<vi>)
      n239 = control-ref of="Queue Array"() -> (w945:refnum<vi>)
      n240 = control-ref of="Queue JSON"() -> (w681:refnum<vi>)
      n241 = control-ref of="Countdown Array"() -> (w984:refnum<vi>)
      n242 = control-ref of="Pressure Limit Tripped Array"() -> (w885:refnum<vi>)
      n243 = control-ref of="Current Locks"() -> (w695:refnum<vi>)
      n244 = control-ref of="Stop Program"() -> (w682:refnum<vi>)
      n245 = control-ref of="Current Valve State"() -> (w700:refnum<vi>)
      n246 = property class="Arr (strict)"(reference=w944) -> ("Value"=w911:refnum<vi>[])  [unwired: 1 in, 2 out]
      n247 = property class="Arr (strict)"(reference=w887) -> ("Value"=w886:refnum<vi>[])  [unwired: 1 in, 2 out]
      n248 = control-ref of="Lock Reentrance Rate"() -> (w741:refnum<vi>)
      n249 = property class="Arr (strict)"(reference=w984) -> ("Value"=w950:refnum<vi>[])  [unwired: 1 in, 2 out]
      n250 = property class="Arr (strict)"(reference=w773) -> ("Value"=w765:refnum<vi>[])  [unwired: 1 in, 2 out]
      n251 = property class="Arr (strict)"(reference=w945) -> ("Value"=w658:refnum<vi>[])  [unwired: 1 in, 2 out]
      n252 = property class="Arr (strict)"(reference=w885) -> ("Value"=w892:refnum<vi>[])  [unwired: 1 in, 2 out]
      n253 = property class="Arr (strict)"(reference=w778) -> ("Value"=w776:refnum<vi>[])  [unwired: 1 in, 2 out]
      n254 = property class="Arr (strict)"(reference=w832) -> (reference out=w831:refnum<vi>, "Value"=w829:refnum<vi>[])  [unwired: 1 in, 1 out]
      n255 = vi-ref "Pressure Read Loop.vi"() -> (w927:refnum<vi>)
      n256 = control-ref of="Debug Mode"() -> (w694:refnum<vi>)
      n257 = control-ref of="Manual Override\nPump Shared Array"() -> (w987:refnum<vi>)
      n258 = Or(x=64 ("options"), y=128 ("options")) -> (x .or. y?=w923:i32)
      n259 = control-ref of="Manual Override\nChamber Array"() -> (w988:refnum<vi>)
      n260 = control-ref of="Default Purge"() -> (w711:refnum<vi>)
      n261 = control-ref of="System Log"() -> (w869:refnum<vi>)
      n262 = local read "Reactor Name"() -> (w676:string)
      n263 = property class="VI"(reference=w927) -> ("Name"=w926:string)  [unwired: 1 in, 2 out]
      n264 = control-ref of="Start Time Array"() -> (w656:refnum<vi>)
      n265 = control-ref of="Save Table Reactor Array"() -> (w980:refnum<vi>)
      n266 = Build Array (concatenate)(w670, w868) -> (w699:refnum<vi>[])
      n267 = control-ref of="Error Trip Cycle Array"() -> (w889:refnum<vi>)
      n268 = control-ref of="Save File Connection Array"() -> (w948:refnum<vi>)
      n269 = control-ref of="Current Cycle Reactor Array"() -> (w947:refnum<vi>)
      n270 = control-ref of="Header Connection txt Array"() -> (w779:refnum<vi>)
      n271 = control-ref of="Pressure Limit"() -> (w891:refnum<vi>)
      n272 = control-ref of="GUID array"() -> (w949:refnum<vi>)
      n273 = local read "Number of Reactors"() -> (w792:i32)
      n274 = control-ref of="Pressure (mTorr) Array"() -> (w929:refnum<vi>)
      n275 = control-ref of="Pressure Graph Array"() -> (w928:refnum<vi>)
      n276 = vi-ref "CountdownTimer.vi"() -> (w958:refnum<vi>)
      n277 = vi-ref "SaveLoadTables.vi"() -> (w978:refnum<vi>)
      n278 = Open VI Reference(type specifier VI Refnum (for type only)=refnum<vi> refnum, vi path=w926, options=w923) -> (vi reference=w922:refnum<vi>, error out=w921:errorcluster)  [unwired: 3 in]
      n279 = property class="Arr (strict)"(reference=w889) -> ("Value"=w888:refnum<vi>[])  [unwired: 1 in, 2 out]
      n280 = property class="Arr (strict)"(reference=w947) -> ("Value"=w910:refnum<vi>[])  [unwired: 1 in, 2 out]
      n281 = vi-ref "Pressure Queue Consumer Loop.vi"() -> (w931:refnum<vi>)
      n282 = property class="Arr (strict)"(reference=w656) -> ("Value"=w660:refnum<vi>[])  [unwired: 1 in, 2 out]
      n283 = property class="Arr (strict)"(reference=w948) -> ("Value"=w909:refnum<vi>[])  [unwired: 1 in, 2 out]
      n284 = local read "Reactor Selector"() -> (w674:T1)
      n285 = property class="Arr (strict)"(reference=w980) -> ("Value"=w979:refnum<vi>[])  [unwired: 1 in, 2 out]
      n286 = property class="Arr (strict)"(reference=w779) -> ("Value"=w775:refnum<vi>[])  [unwired: 1 in, 2 out]
      n287 = local read "Number of Shared Lines"() -> (w675:i32)
      n288 = vi-ref "Start Process.vi"() -> (w807:refnum<vi>)
      n289 = Or(x=64 ("options"), y=128 ("options")) -> (x .or. y?=w974:i32)
      n290 = property class="Arr (strict)"(reference=w928) -> ("Value"=w913:refnum<vi>[])  [unwired: 1 in, 2 out]
      n291 = Or(x=64 ("options"), y=128 ("options")) -> (x .or. y?=w935:i32)
      n292 = control-ref of="Queue System"() -> (w696:refnum<vi>)
      n293 = property class="VI"(reference=w958) -> ("Name"=w959:string)  [unwired: 1 in, 2 out]
      n294 = invoke class="VI (strict)" method="Populate Async Call Pool"(reference=w922, error in=w921, "MinimumSize"=1 ("Minimum Size")) -> (reference out=w917:refnum<vi>, error out=w916:errorcluster)  [unwired: 2 in, 3 out]
      n295 = property class="VI"(reference=w978) -> ("Name"=w977:string)  [unwired: 1 in, 2 out]
      n296 = property class="Arr (strict)"(reference=w929) -> ("Value"=w893:refnum<vi>[])  [unwired: 1 in, 2 out]
      n297 = property class="Arr (strict)"(reference=w949) -> ("Value"=w659:refnum<vi>[])  [unwired: 1 in, 2 out]
      n298 = Or(x=64 ("options"), y=128 ("options")) -> (x .or. y?=w962:i32)
      n299 = Or(x=64 ("options"), y=128 ("options")) -> (x .or. y?=w803:i32)
      n300 = property class="VI"(reference=w931) -> ("Name"=w932:string)  [unwired: 1 in, 2 out]
      n301 = local read "N2 Valves"() -> (w698:i32[])
      n302 = local read "Pump Valves"() -> (w697:i32[])
      n303 = property class="Arr (strict)"(reference=w987) -> ("Value"=w986:refnum<vi>[])  [unwired: 1 in, 2 out]
      n304 = property class="Arr (strict)"(reference=w988) -> ("Value"=w985:refnum<vi>[])  [unwired: 1 in, 2 out]
      n305 = property class="VI"(reference=w807) -> ("Name"=w806:string)  [unwired: 1 in, 2 out]
      n306 = Build Array (concatenate)(w829, w828) -> (w818:refnum<vi>[])
      n307 = control-ref of="Username Array"() -> (w770:refnum<vi>)
      n308 = Open VI Reference(type specifier VI Refnum (for type only)=refnum<vi> refnum, vi path=w959, options=w962) -> (vi reference=w963:refnum<vi>, error out=w964:errorcluster)  [unwired: 3 in]
      n309 = Open VI Reference(type specifier VI Refnum (for type only)=refnum<vi> refnum, vi path=w977, options=w974) -> (vi reference=w973:refnum<vi>, error out=w970:errorcluster)  [unwired: 3 in]
      n310 = Open VI Reference(type specifier VI Refnum (for type only)=refnum<vi> refnum, vi path=w932, options=w935) -> (vi reference=w936:refnum<vi>, error out=w939:errorcluster)  [unwired: 3 in]
      n311 = Open VI Reference(type specifier VI Refnum (for type only)=refnum<vi> refnum, vi path=w806, options=w803) -> (vi reference=w802:refnum<vi>, error out=w801:errorcluster)  [unwired: 3 in]
      n312 = control-ref of="Current Cycle Reactor Array"() -> (w733:refnum<vi>)
      n313 = property class="Arr (strict)"(reference=w770) -> ("Value"=w769:refnum<vi>[])  [unwired: 1 in, 2 out]
      n314 = Build Array (concatenate)(w986, w985) -> (w819:refnum<vi>[])
      n315 = invoke class="VI Interface Type 8" method="Populate Async Call Pool"(reference=w963, error in=w964, "MinimumSize"=w792) -> (reference out=w956:refnum<vi>, error out=w955:errorcluster)  [unwired: 2 in, 3 out]
      n316 = invoke class="VI (strict)" method="Populate Async Call Pool"(reference=w973, error in=w970, "MinimumSize"=w792) -> (reference out=w972:refnum<vi>, error out=w969:errorcluster)  [unwired: 2 in, 3 out]
      n317 = control-ref of="Time Left Array"() -> (w726:refnum<vi>)
      n318 = invoke class="VI (strict)" method="Populate Async Call Pool"(reference=w936, error in=w939, "MinimumSize"=w792) -> (reference out=w937:refnum<vi>, error out=w940:errorcluster)  [unwired: 2 in, 3 out]
      n319 = local read "Number of Shared Lines"() -> (w683:i32)
      n320 = invoke class="VI (strict)" method="Populate Async Call Pool"(reference=w802, error in=w801, "MinimumSize"=w792) -> (reference out=w783:refnum<vi>, error out=w782:errorcluster)  [unwired: 2 in, 3 out]
      n321 = property class="Arr (strict)"(reference=w733) -> ("Value"=w732:refnum<vi>[])  [unwired: 1 in, 2 out]
      n322 = call-by-ref "Start Asynchronous Call"(reference=w917, error in=w916, "Pressure Graph Array Ref"=w913, "Pressure (mTorr) Array Ref"=w893, "Number of Reactors"=w792, "Logging Data Array Ref"=w911, "Pressure Scale Array"=w690, "Pressure Voltage\nCorrect Array"=w691, "Queue Array Ref"=w658, "Debug Mode"=w694, "Reactor Selector"=w673, "Stop Program"=w682, "Current Cycle Reactor X"=w661, "Start Time Reactor X"=w662, "GUID X"=w659) -> (reference out=w915:refnum<vi>, error out=w914:errorcluster)  [unwired: 15 in]
      n323 = control-ref of="Save JSON log Connection"() -> (w679:refnum<vi>)
      n324 = control-ref of="date on current file"() -> (w680:refnum<vi>)
      n325 = property class="Arr (strict)"(reference=w726) -> ("Value"=w724:refnum<vi>[])  [unwired: 1 in, 2 out]
      n326 = local read "Pump Valves"() -> (w747:i32[])
      n327 = Close Reference(reference=w915, error in (no error)=w914) -> (error out=w920:errorcluster)
      n328 = control-ref of="Experimental Details Array"() -> (w771:refnum<vi>)
      n329 = vi-ref "System Log Consumer Loop.vi"() -> (w878:refnum<vi>)
      n330 = vi-ref "Manual Override Loop.vi"() -> (w701:refnum<vi>)
      n331 = Or(x=64 ("options"), y=128 ("options")) -> (x .or. y?=w882:i32)
      n332 = control-ref of="Table Position Reactor Array"() -> (w735:refnum<vi>)
      n333 = property class="Arr (strict)"(reference=w771) -> ("Value"=w768:refnum<vi>[])  [unwired: 1 in, 2 out]
      n334 = property class="VI"(reference=w878) -> ("Name"=w879:string)  [unwired: 1 in, 2 out]
      n335 = local read "N2 Valves"() -> (w748:i32[])
      n336 = control-ref of="Completion Array"() -> (w727:refnum<vi>)
      n337 = call <vilib>:"Simple Error Handler.vi"("type of dialog (OK msg:1)"=w919, "error in (no error)"=w920) -> ()  [unwired: 3 in, 5 out]
      n338 = vi-ref "Emergency Process Stop.vi"() -> (w834:refnum<vi>)
      n339 = property class="VI"(reference=w701) -> ("Name"=w702:string)  [unwired: 1 in, 2 out]
      n340 = vi-ref "Manual Override Button Enable Disable Shared.vi"() -> (w853:refnum<vi>)
      n341 = local read "System Constants"() -> (w684:T4)
      n342 = property class="Arr (strict)"(reference=w735) -> ("Value"=w734:refnum<vi>[])  [unwired: 1 in, 2 out]
      n343 = vi-ref "System Log JSON Consumer Loop.vi"() -> (w817:refnum<vi>)
      n344 = vi-ref "Pressure Limit Checker.vi"() -> (w907:refnum<vi>)
      n345 = property class="Arr (strict)"(reference=w727) -> ("Value"=w725:refnum<vi>[])  [unwired: 1 in, 2 out]
      n346 = Open VI Reference(type specifier VI Refnum (for type only)=refnum<vi> refnum, vi path=w879, options=w882) -> (vi reference=w876:refnum<vi>, error out=w875:errorcluster)  [unwired: 3 in]
      n347 = vi-ref "Manual Override Button Enable Disable Reactor.vi"() -> (w860:refnum<vi>)
      n348 = property class="VI"(reference=w834) -> ("Name"=w835:string)  [unwired: 1 in, 2 out]
      n349 = local read "Valves on Shared 1"() -> (w762:i32)
      n350 = Or(x=64 ("options"), y=128 ("options")) -> (x .or. y?=w903:i32)
      n351 = property class="VI"(reference=w853) -> ("Name"=w852:string)  [unwired: 1 in, 2 out]
      n352 = Open VI Reference(type specifier VI Refnum (for type only)=refnum<vi> refnum, vi path=w702) -> (vi reference=w703:refnum<vi>, error out=w704:errorcluster)  [unwired: 4 in]
      n353 = control-ref of="Time Elapsed Array"() -> (w774:refnum<vi>)
      n354 = invoke class="VI Interface Type 4" method="Populate Async Call Pool"(reference=w876, error in=w875, "MinimumSize"=1 ("Minimum Size")) -> (reference out=w873:refnum<vi>, error out=w872:errorcluster)  [unwired: 2 in, 3 out]
      n355 = property class="VI"(reference=w817) -> ("Name"=w816:string)  [unwired: 1 in, 2 out]
      n356 = property class="VI"(reference=w907) -> ("Name"=w906:string)  [unwired: 1 in, 2 out]
      n357 = Or(x=64 ("options"), y=128 ("options")) -> (x .or. y?=w864:i32)
      n358 = vi-ref "Stop Process.vi"() -> (w794:refnum<vi>)
      n359 = property class="VI"(reference=w860) -> ("Name"=w861:string)  [unwired: 1 in, 2 out]
      n360 = Open VI Reference(type specifier VI Refnum (for type only)=refnum<vi> refnum, vi path=w835) -> (vi reference=w836:refnum<vi>, error out=w837:errorcluster)  [unwired: 4 in]
      n361 = vi-ref "Run Process.vi"() -> (w756:refnum<vi>)
      n362 = call-by-ref "?"(reference=w703, error in=w704, "Current Valve State Array"=w700, "Manual Valve Array"=w699, "Stop Process"=w682, "System Queue"=w696, "N2 Valves"=w698, "JSON Queue"=w681, "Pump Valves"=w697, "Locks (-)"=w695, "Valves Per Reactor"=w671, "Debug Mode"=w694, "Number of Reactors"=w672, "Reactor Name"=w677, "Reactor Selector"=w673, "Number of Shared Lines"=w685) -> (reference out=w705:refnum<vi>, error out=w706:errorcluster)  [unwired: 6 in]
      n363 = control-ref of="Start Stop Reactor Array"() -> (w739:refnum<vi>)
      n364 = vi-ref "Default Behavior.vi"() -> (w716:refnum<vi>)
      n365 = Open VI Reference(type specifier VI Refnum (for type only)=refnum<vi> refnum, vi path=w852) -> (vi reference=w851:refnum<vi>, error out=w850:errorcluster)  [unwired: 4 in]
      n366 = vi-ref "Manual Override Lock Control.vi"() -> (w827:refnum<vi>)
      n367 = Or(x=64 ("options"), y=128 ("options")) -> (x .or. y?=w798:i32)
      n368 = property class="Arr (strict)"(reference=w774) -> ("Value"=w766:refnum<vi>[])  [unwired: 1 in, 2 out]
      n369 = control-ref of="Current Cycle Display Array"() -> (w729:refnum<vi>)
      n370 = Open VI Reference(type specifier VI Refnum (for type only)=refnum<vi> refnum, vi path=w816) -> (vi reference=w815:refnum<vi>, error out=w811:errorcluster)  [unwired: 4 in]
      n371 = property class="VI"(reference=w794) -> ("Name"=w795:string)  [unwired: 1 in, 2 out]
      n372 = Or(x=64 ("options"), y=128 ("options")) -> (x .or. y?=w753:i32)
      n373 = Open VI Reference(type specifier VI Refnum (for type only)=refnum<vi> refnum, vi path=w906, options=w903) -> (vi reference=w902:refnum<vi>, error out=w901:errorcluster)  [unwired: 3 in]
      n374 = local read "Valves on Shared 2"() -> (w763:i32)
      n375 = property class="VI"(reference=w756) -> ("Name"=w755:string)  [unwired: 1 in, 2 out]
      n376 = call-by-ref "?"(reference=w851, error in=w850, "Stop Program"=w682, "Valves on Shared Lines"=w843, "Pump Shared Lock Claimed Array"=w831, "Shared Manual Valve Array"=w844) -> (reference out=w849:refnum<vi>, error out=w848:errorcluster)
      n377 = Close Reference(reference=w705, error in (no error)=w706) -> (error out=w709:errorcluster)
      n378 = property class="VI"(reference=w716) -> ("Name"=w717:string)  [unwired: 1 in, 2 out]
      n379 = property class="Arr (strict)"(reference=w739) -> ("Value"=w736:refnum<vi>[])  [unwired: 1 in, 2 out]
      n380 = property class="VI"(reference=w827) -> ("Name"=w826:string)  [unwired: 1 in, 2 out]
      n381 = Open VI Reference(type specifier VI Refnum (for type only)=refnum<vi> refnum, vi path=w861, options=w864) -> (vi reference=w865:refnum<vi>, error out=w866:errorcluster)  [unwired: 3 in]
      n382 = property class="Arr (strict)"(reference=w729) -> ("Value"=w728:refnum<vi>[])  [unwired: 1 in, 2 out]
      n383 = invoke class="VI Interface Type 5" method="Populate Async Call Pool"(reference=w902, error in=w901, "MinimumSize"=w792) -> (reference out=w895:refnum<vi>, error out=w894:errorcluster)  [unwired: 2 in, 3 out]
      n384 = call-by-ref "Start Asynchronous Call"(reference=w873, error in=w872, "Stop Program"=w682, "System Queue"=w696, "System Visual Log"=w869) -> (reference out=w871:refnum<vi>, error out=w870:errorcluster)
      n385 = Open VI Reference(type specifier VI Refnum (for type only)=refnum<vi> refnum, vi path=w795, options=w798) -> (vi reference=w799:refnum<vi>, error out=w800:errorcluster)  [unwired: 3 in]
      n386 = Close Reference(reference=w849, error in (no error)=w848) -> (error out=w845:errorcluster)
      n387 = invoke class="VI Interface Type 3" method="Populate Async Call Pool"(reference=w865, error in=w866, "MinimumSize"=w792) -> (reference out=w855:refnum<vi>, error out=w854:errorcluster)  [unwired: 2 in, 3 out]
      n388 = control-ref of="ALD Sequence for Reactor Array"() -> (w772:refnum<vi>)
      n389 = Open VI Reference(type specifier VI Refnum (for type only)=refnum<vi> refnum, vi path=w717) -> (vi reference=w718:refnum<vi>, error out=w715:errorcluster)  [unwired: 4 in]
      n390 = call <vilib>:"Simple Error Handler.vi"("type of dialog (OK msg:1)"=w708, "error in (no error)"=w709) -> ()  [unwired: 3 in, 5 out]
      n391 = Open VI Reference(type specifier VI Refnum (for type only)=refnum<vi> refnum, vi path=w826) -> (vi reference=w825:refnum<vi>, error out=w714:errorcluster)  [unwired: 4 in]
      n392 = local read "Reactor Name"() -> (w678:string)
      n393 = call-by-ref "?"(reference=w836, error in=w837, "Emergency Process Stop"=w833, "Start Stop Reactor Array"=w830, "Reactor Name"=w678, "Reactor Selector"=w673, "Current Valve State"=w700, "System Queue"=w696, "System JSON Queue"=w681, "Pump Valves"=w697, "Debug Mode"=w694, "Stop Program"=w682) -> (reference out=w838:refnum<vi>, error out=w839:errorcluster)  [unwired: 6 in]
      n394 = call-by-ref "?"(reference=w815, error in=w811, "Reactor Name"=w678, "Stop Program"=w682, "date on current file"=w680, "Queue JSON"=w681, "Save JSON log Connection"=w679) -> (reference out=w814:refnum<vi>, error out=w810:errorcluster)
      n395 = Close Reference(reference=w838, error in (no error)=w839) -> (error out=w842:errorcluster)
      n396 = Close Reference(reference=w814, error in (no error)=w810) -> (error out=w809:errorcluster)
      n397 = Open VI Reference(type specifier VI Refnum (for type only)=refnum<vi> refnum, vi path=w755, options=w753) -> (vi reference=w752:refnum<vi>, error out=w751:errorcluster)  [unwired: 3 in]
      n398 = control-ref of="System Idle Array"() -> (w738:refnum<vi>)
      n399 = call <vilib>:"Simple Error Handler.vi"("type of dialog (OK msg:1)"=w841, "error in (no error)"=w842) -> ()  [unwired: 3 in, 5 out]
      n400 = invoke class="VI (strict)" method="Populate Async Call Pool"(reference=w799, error in=w800, "MinimumSize"=w792) -> (reference out=w781:refnum<vi>, error out=w780:errorcluster)  [unwired: 2 in, 3 out]
      n401 = Close Reference(reference=w871, error in (no error)=w870) -> (error out=w883:errorcluster)
      n402 = control-ref of="ALD Sequence for Reactor Array"() -> (w731:refnum<vi>)
      n403 = local read "Valves Per Reactor"() -> (w764:i32)
      n404 = call-by-ref "?"(reference=w718, error in=w715, "Start Stop Reactor Array"=w713, "System Idle Array"=w712, "Default Purge"=w711, "Current Valve State"=w700, "Current Locks"=w695, "Reactor Name"=w676, "Number of Reactors"=w672, "Stop Program"=w682, "Valves Per Reactor"=w671, "Debug Mode"=w694, "Lock Reentrance Rate"=w710, "Queue System"=w696, "Pump Valves"=w697, "Queue JSON Object"=w681, "Number of Shared Lines"=w675, "Reactor Selector"=w674) -> (reference out=w719:refnum<vi>, error out=w720:errorcluster)  [unwired: 4 in]
      n405 = call-by-ref "?"(reference=w825, error in=w714, "Buttons to Claim Manual Control Lock"=w819, "Reactor Name"=w676, "Indicators for Manual Control Lock Claimed"=w818, "Current Locks"=w695, "Lock Reentrance Rate"=w710, "Queue System"=w696, "JSON Queue"=w681, "Stop Program"=w682) -> (reference out=w824:refnum<vi>, error out=w823:errorcluster)  [unwired: 8 in]
      n406 = call <vilib>:"Simple Error Handler.vi"("type of dialog (OK msg:1)"=w846, "error in (no error)"=w845) -> ()  [unwired: 3 in, 5 out]
      n407 = property class="Arr (strict)"(reference=w772) -> ("Value"=w767:refnum<vi>[])  [unwired: 1 in, 2 out]
      n408 = invoke class="VI (strict)" method="Populate Async Call Pool"(reference=w752, error in=w751) -> (reference out=w750:refnum<vi>, error out=w749:errorcluster)  [unwired: 3 in, 3 out]
      n409 = call <vilib>:"Simple Error Handler.vi"("type of dialog (OK msg:1)"=w812, "error in (no error)"=w809) -> ()  [unwired: 3 in, 5 out]
      n410 = property class="Arr (strict)"(reference=w738) -> ("Value"=w737:refnum<vi>[])  [unwired: 1 in, 2 out]
      n411 = Close Reference(reference=w719, error in (no error)=w720) -> (error out=w723:errorcluster)
      n412 = call <vilib>:"Simple Error Handler.vi"("type of dialog (OK msg:1)"=w884, "error in (no error)"=w883) -> ()  [unwired: 3 in, 5 out]
      n413 = Close Reference(reference=w824, error in (no error)=w823) -> (error out=w820:errorcluster)
      n414 = property class="Arr (strict)"(reference=w731) -> ("Value"=w730:refnum<vi>[])  [unwired: 1 in, 2 out]
      n415 = call <vilib>:"Simple Error Handler.vi"("type of dialog (OK msg:1)"=w722, "error in (no error)"=w723) -> ()  [unwired: 3 in, 5 out]
      n416 = call <vilib>:"Simple Error Handler.vi"("type of dialog (OK msg:1)"=w821, "error in (no error)"=w820) -> ()  [unwired: 3 in, 5 out]
      n417 = control-ref of="Experimental Details for Reactor Array"() -> (w666:refnum<vi>)
      n418 = control-ref of="Username for Reactor Array"() -> (w665:refnum<vi>)
      n419 = control-ref of="ALD Sequence for Reactor Array"() -> (w668:refnum<vi>)
      n420 = property class="Arr (strict)"(reference=w666) -> ("Value"=w664:refnum<vi>[])  [unwired: 1 in, 2 out]
      n421 = property class="Arr (strict)"(reference=w665) -> ("Value"=w663:refnum<vi>[])  [unwired: 1 in, 2 out]
      n422 = property class="Arr (strict)"(reference=w668) -> ("Value"=w667:refnum<vi>[])  [unwired: 1 in, 2 out]
      n423 = for {
        N: w792 -> [w1047]
        tunnel: w983 -> [w1052] mode=indexing
        tunnel: w981 -> [w1069] mode=indexing
        tunnel: w979 -> [w1104] mode=indexing
        shift-right: [w1103] -> w971
        shift-left: w972 -> [w1106]
        shift-right: [w1102] -> w968
        shift-left: w969 -> [w1105]
        shift-right: [w1099] -> w954
        shift-left: w956 -> [w1101]
        shift-right: [w1098] -> w953
        shift-left: w955 -> [w1100]
        tunnel: w950 -> [w1044] mode=indexing
        shift-right: [w1096] -> w938
        shift-left: w937 -> [w1094]
        shift-right: [w1097] -> w941
        shift-left: w940 -> [w1095]
        tunnel: w909 -> [w1065] mode=indexing
        tunnel: w662 -> [w1093] mode=indexing
        tunnel: w658 -> [w1062] mode=indexing
        tunnel: w910 -> [w1092] mode=indexing
        tunnel: w908 -> [w1064] mode=indexing
        tunnel: w911 -> [w1067] mode=indexing
        tunnel: w659 -> [w1057] mode=indexing
        tunnel: w682 -> [w1021]
        shift-right: [w1089] -> w897
        shift-left: w895 -> [w1090]
        shift-right: [w1088] -> w896
        shift-left: w894 -> [w1091]
        tunnel: w893 -> [w1042] mode=indexing
        tunnel: w892 -> [w1087] mode=indexing
        tunnel: w891 -> [w1086]
        tunnel: w661 -> [w1085] mode=indexing
        tunnel: w888 -> [w1084] mode=indexing
        tunnel: w886 -> [w1083] mode=indexing
        tunnel: w696 -> [w1082]
        tunnel: w681 -> [w1037]
        shift-right: [w1081] -> w857
        shift-left: w855 -> [w1079]
        shift-right: [w1080] -> w856
        shift-left: w854 -> [w1078]
        tunnel: w831 -> [w1018]
        tunnel: w828 -> [w1017] mode=indexing
        shift-right: [w1076] -> w788
        shift-left: w783 -> [w1074]
        shift-right: [w1077] -> w789
        shift-left: w782 -> [w1075]
        shift-right: [w1071] -> w787
        shift-left: w781 -> [w1073]
        shift-right: [w1070] -> w786
        shift-left: w780 -> [w1072]
        tunnel: w777 -> [w1068] mode=indexing
        tunnel: w776 -> [w1066] mode=indexing
        tunnel: w775 -> [w1063] mode=indexing
        tunnel: w696 -> [w1036]
        tunnel: w695 -> [w1027]
        tunnel: w710 -> [w1061]
        tunnel: w660 -> [w1056] mode=indexing
        tunnel: w769 -> [w1060] mode=indexing
        tunnel: w768 -> [w1059] mode=indexing
        tunnel: w767 -> [w1058] mode=indexing
        tunnel: w766 -> [w1055] mode=indexing
        tunnel: w765 -> [w1045] mode=indexing
        tunnel: w694 -> [w1038]
        tunnel: w700 -> [w1026]
        tunnel: w764 -> [w1012]
        tunnel: w763 -> [w1054]
        tunnel: w762 -> [w1046]
        tunnel: w697 -> [w1053]
        shift-right: [w1050] -> w758
        shift-left: w750 -> [w1048]
        shift-right: [w1051] -> w759
        shift-left: w749 -> [w1049]
        tunnel: w748 -> [_]
        tunnel: w747 -> [_]
        tunnel: w745 -> [w1043] mode=indexing
        tunnel: w743 -> [w1041] mode=indexing
        tunnel: w742 -> [w1040]
        tunnel: w741 -> [w1039]
        tunnel: w737 -> [w1035] mode=indexing
        tunnel: w736 -> [w1034] mode=indexing
        tunnel: w734 -> [w1033] mode=indexing
        tunnel: w732 -> [w1032] mode=indexing
        tunnel: w730 -> [w1031] mode=indexing
        tunnel: w728 -> [w1030] mode=indexing
        tunnel: w725 -> [w1029] mode=indexing
        tunnel: w724 -> [w1028] mode=indexing
        tunnel: w682 -> [w1016]
        tunnel: w685 -> [w1015]
        tunnel: w677 -> [w1025]
        tunnel: w678 -> [w1022]
        tunnel: w684 -> [w1024]
        tunnel: w683 -> [w1023]
        tunnel: w673 -> [w1020]
        tunnel: w669 -> [w1019]
        tunnel: w667 -> [w1010] mode=indexing
        tunnel: w664 -> [w1008] mode=indexing
        tunnel: w663 -> [w1009] mode=indexing
        tunnel: w660 -> [w1007] mode=indexing
        tunnel: w659 -> [w1006] mode=indexing
        tunnel: w658 -> [w1005] mode=indexing
        i -> [w1014]
        n424 = call-by-ref "Start Asynchronous Call"(reference=w1101, error in=w1100, "Stop Program"=w1021, "Countdown X"=w1044) -> (reference out=w1099:refnum<vi>, error out=w1098:errorcluster)  [unwired: 1 in]
        n425 = call-by-ref "Start Asynchronous Call"(reference=w1074, error in=w1075, "Stop / Start Reactor X"=w1052, "System Idle Pressure X"=w1068, "Reactor Number"=w1014, "Logging Data X"=w1067, "Save File Connection X"=w1065, "Save File JSON Connection X"=w1064, "Header Connection txt Array"=w1063, "Queue Reactor X"=w1062, "Start Time Reactor X"=w1056, "Queue System"=w1036, "Username X"=w1060, "Current Locks"=w1027, "Experimental Details X"=w1059, "System JSON Queue"=w1037, "ALD Sequence for Reactor X"=w1058, "Stop Program"=w1021, "Number of Shared Lines"=w1023, "Lock Reentrance Rate"=w1061, "GUID X"=w1057, "Reactor Name"=w1022) -> (reference out=w1076:refnum<vi>, error out=w1077:errorcluster)  [unwired: 8 in]
        n426 = call-by-ref "Start Asynchronous Call"(reference=w1094, error in=w1095, "Save File Connection X"=w1065, "Start Time Reactor X"=w1093, "Queue Reactor X"=w1062, "Current Cycle Reactor X"=w1092, "Save File JSON Connection X"=w1064, "Logging Data X"=w1067, "Reactor Name"=w1025, "Reactor Number"=w1014, "Stop Program"=w1016) -> (reference out=w1096:refnum<vi>, error out=w1097:errorcluster)  [unwired: 11 in]
        n427 = call-by-ref "Start Asynchronous Call"(reference=w1090, error in=w1091, "Pressure\nLimit\nTripped X"=w1087, "Pressure (mTorr) X"=w1042, "Pressure Limit"=w1086, "Stop / Start Reactor X"=w1052, "Current Cycle Reactor X"=w1085, "Error Trip Cycle X"=w1084, "System Queue"=w1082, "Error Trip Time X"=w1083, "System JSON Queue"=w1037, "Reactor Number"=w1014, "Reactor Name"=w1022, "Stop Program"=w1021) -> (reference out=w1089:refnum<vi>, error out=w1088:errorcluster)  [unwired: 8 in]
        n428 = call-by-ref "Start Asynchronous Call"(reference=w1073, error in=w1072, "Stop / Start Reactor X"=w1052, "System Idle Pressure X"=w1068, "Reactor Number"=w1014, "Logging Data X"=w1067, "Countdown X"=w1066, "Save File Connection X"=w1065, "Save File JSON Connection X"=w1064, "Header Connection txt X"=w1063, "Valves on Shared 1"=w1046, "Stop Program"=w1021, "Valves on Shared 2"=w1054, "Queue System"=w1036, "Number of Reactors"=w1047, "System JSON Queue"=w1037, "Valves Per Reactor"=w1012, "Current Locks"=w1027, "Pump Valves"=w1053, "Current Valve State X"=w1026, "Reactor Name"=w1022, "Debug Mode X"=w1038, "Wait Before Start (s) X"=w1045, "Number of Shared Lines"=w1023, "Start Time Reactor X"=w1056, "Reactor Selector"=w1020, "Time Elapsed X"=w1055, "GUID X"=w1057) -> (reference out=w1071:refnum<vi>, error out=w1070:errorcluster)  [unwired: 2 in]
        n429 = Increment(x=w1014) -> (x+1=w1013:i32)
        n430 = call-by-ref "Start Asynchronous Call"(reference=w1079, error in=w1078, "Number of Shared Lines"=w1015, "Reactor Number"=w1013, "Valves Per Reactor"=w1012, "Stop Program"=w1016, "Chamber Lock Claimed X"=w1017, "Pump Shared Lock Claimed Array"=w1018, "Manual Valve Array"=w1019) -> (reference out=w1081:refnum<vi>, error out=w1080:errorcluster)  [unwired: 1 in]
        n431 = call-by-ref "Start Asynchronous Call"(reference=w1048, error in=w1049, "Time Left X"=w1028, "Completion X"=w1029, "Current Cycle Display X"=w1030, "ALD Sequence for Reactor X"=w1031, "Current Cycle Reactor X"=w1032, "Table Position Reactor X"=w1033, "Stop / Start Reactor X"=w1034, "System Idle X"=w1035, "Reactor Number (Base 0)"=w1014, "Stop Program"=w1021, "Start Time Reactor X"=w1007, "System Queue"=w1036, "System Constants"=w1024, "System JSON Queue"=w1037, "Reactor Selector"=w1020, "Current Locks"=w1027, "GUID X"=w1006, "Current Valve State"=w1026, "Queue Reactor X"=w1005, "Debug Mode"=w1038, "Wait Before Start (s) X"=w1045, "Timer Reactor X"=w1043, "Countdown X"=w1044, "Pressure (mTorr) X"=w1042, "Recorded Pressure X"=w1041, "Lock Reentrance Rate"=w1039, "Valve Close Delay"=w1040) -> (reference out=w1050:refnum<vi>, error out=w1051:errorcluster)  [unwired: 1 in]
        n432 = Bundle("ALD Sequence for Reactor 6"=w1010, "Username 6"=w1009, "Experimental Details 6"=w1008) -> (w1011:T6)  [unwired: 1 in]
        n433 = call-by-ref "Start Asynchronous Call"(reference=w1106, error in=w1105, "Stop Program"=w1021, "Reactor Data"=w1011, "Stop / Start Reactor X"=w1052, "Save Table Reactor X"=w1104, "Load Table Reactor X"=w1069) -> (reference out=w1103:refnum<vi>, error out=w1102:errorcluster)  [unwired: 1 in]
      }
      n434 = Close Reference(reference=w954, error in (no error)=w953) -> (error out=w951:errorcluster)
      n435 = Close Reference(reference=w971, error in (no error)=w968) -> (error out=w967:errorcluster)
      n436 = Close Reference(reference=w857, error in (no error)=w856) -> (error out=w858:errorcluster)
      n437 = Close Reference(reference=w897, error in (no error)=w896) -> (error out=w899:errorcluster)
      n438 = control-ref of="Running Reactor\nIndicator Array"() -> (w687:refnum<vi>)
      n439 = Close Reference(reference=w938, error in (no error)=w941) -> (error out=w942:errorcluster)
      n440 = call <vilib>:"Simple Error Handler.vi"("type of dialog (OK msg:1)"=w966, "error in (no error)"=w967) -> ()  [unwired: 3 in, 5 out]
      n441 = call <vilib>:"Simple Error Handler.vi"("type of dialog (OK msg:1)"=w859, "error in (no error)"=w858) -> ()  [unwired: 3 in, 5 out]
      n442 = call <vilib>:"Simple Error Handler.vi"("type of dialog (OK msg:1)"=w898, "error in (no error)"=w899) -> ()  [unwired: 3 in, 5 out]
      n443 = call <vilib>:"Simple Error Handler.vi"("type of dialog (OK msg:1)"=w943, "error in (no error)"=w942) -> ()  [unwired: 3 in, 5 out]
      n444 = call <vilib>:"Simple Error Handler.vi"("type of dialog (OK msg:1)"=w952, "error in (no error)"=w951) -> ()  [unwired: 3 in, 5 out]
      n445 = property class="Arr (strict)"(reference=w687) -> ("Value"=w686:refnum<vi>[])  [unwired: 1 in, 2 out]
      n446 = control-ref of="Valve Indicator Array"() -> (w689:refnum<vi>)
      n447 = Close Reference(reference=w788, error in (no error)=w789) -> (error out=w791:errorcluster)
      n448 = Close Reference(reference=w787, error in (no error)=w786) -> (error out=w784:errorcluster)
      n449 = property class="Arr (strict)"(reference=w689) -> ("Value"=w688:refnum<vi>[])  [unwired: 1 in, 2 out]
      n450 = Close Reference(reference=w758, error in (no error)=w759) -> (error out=w761:errorcluster)
      n451 = call <vilib>:"Simple Error Handler.vi"("type of dialog (OK msg:1)"=w790, "error in (no error)"=w791) -> ()  [unwired: 3 in, 5 out]
      n452 = call <vilib>:"Simple Error Handler.vi"("type of dialog (OK msg:1)"=w785, "error in (no error)"=w784) -> ()  [unwired: 3 in, 5 out]
      n453 = while {
        tunnel: w686 -> [w993]
        stop <- w990 stop-if-true
        n454 = control-ref of="Start Stop Reactor Array"() -> (w994:refnum<vi>)
        n455 = property class="Arr (strict)"(reference=w994) -> ("Value"=w992:refnum<vi>[])  [unwired: 1 in, 2 out]
        n456 = for {
          tunnel: w993 -> [w997] mode=indexing
          tunnel: w992 -> [w996] mode=indexing
          n457 = property class="Bool (strict)"(reference=w996) -> ("Value"=w995:bool)  [unwired: 1 in, 2 out]
          n458 = property class="Bool (strict)"(reference=w997, "Value"=w995) -> ()  [unwired: 1 in, 2 out]
        }
        n459 = local read "Stop Program"() -> (w990:bool)
        n460 = Wait (ms)(milliseconds to wait=u32 250) -> ()  [unwired: 1 out]
      }
      n461 = call <vilib>:"Simple Error Handler.vi"("type of dialog (OK msg:1)"=w760, "error in (no error)"=w761) -> ()  [unwired: 3 in, 5 out]
      n462 = while {
        tunnel: w688 -> [w1002]
        stop <- w998 stop-if-true
        n463 = control-ref of="Current Valve State"() -> (w1000:refnum<vi>)
        n464 = Wait (ms)(milliseconds to wait=u32 250) -> ()  [unwired: 1 out]
        n465 = property class="Arr (strict)"(reference=w1000) -> ("Value"=w999:bool[])  [unwired: 1 in, 2 out]
        n466 = for {
          tunnel: w1002 -> [w1004] mode=indexing
          tunnel: w999 -> [w1003] mode=indexing
          n467 = property class="Bool (strict)"(reference=w1004, "Value"=w1003) -> ()  [unwired: 1 in, 2 out]
        }
        n468 = local read "Stop Program"() -> (w998:bool)
      }
    }
    frame #4 {
      n469 = local write "Stop Program"(FALSE ("Stop Program")) -> ()
    }
  }
  n470 = Obtain Queue(element data type=w81) -> (queue out=→"Queue Reactor 1":refnum<queue>)  [unwired: 4 in, 2 out]
  n471 = Obtain Queue(element data type=w81) -> (queue out=→"Queue Reactor 2":refnum<queue>)  [unwired: 4 in, 2 out]
  n472 = Obtain Queue(element data type=w81) -> (queue out=→"Queue Reactor 3":refnum<queue>)  [unwired: 4 in, 2 out]
  n473 = Obtain Queue(element data type=w81) -> (queue out=→"Queue Reactor 4":refnum<queue>)  [unwired: 4 in, 2 out]
  n474 = Obtain Queue(element data type=w81) -> (queue out=→"Queue Reactor 5":refnum<queue>)  [unwired: 4 in, 2 out]
  n475 = Obtain Queue(element data type=w81) -> (queue out=→"Queue Reactor 6":refnum<queue>)  [unwired: 4 in, 2 out]
  n476 = Obtain Queue(element data type=w81) -> (queue out=→"Queue System":refnum<queue>)  [unwired: 4 in, 2 out]
  n477 = Obtain Queue(element data type=w81) -> (queue out=→"Queue JSON Object":refnum<queue>)  [unwired: 4 in, 2 out]
  n478 = control-ref of="Last Cycle Temp\nRead Success"() -> (w261:refnum<vi>)
  n479 = control-ref of="Last Cycle Temp\nRead Success 2"() -> (w259:refnum<vi>)
  n480 = control-ref of="Last Cycle Temp\nRead Success 3"() -> (w260:refnum<vi>)
  n481 = control-ref of="Last Cycle Temp\nRead Success 4"() -> (w258:refnum<vi>)
  n482 = control-ref of="Last Cycle Temp\nRead Success 5"() -> (w257:refnum<vi>)
  n483 = control-ref of="Last Cycle Temp\nRead Success 6"() -> (w256:refnum<vi>)
  n484 = control-ref of="Local Connection JSON 1"() -> (w90:refnum<vi>)
  n485 = control-ref of="Local Connection JSON 2"() -> (w85:refnum<vi>)
  n486 = control-ref of="Local Connection JSON 3"() -> (w89:refnum<vi>)
  n487 = control-ref of="Local Connection JSON 4"() -> (w88:refnum<vi>)
  n488 = control-ref of="Local Connection JSON 5"() -> (w87:refnum<vi>)
  n489 = control-ref of="Local Connection JSON 6"() -> (w86:refnum<vi>)
  n490 = control-ref of="Pump\nLock Claimed"() -> (w250:refnum<vi>)
  n491 = control-ref of="Shared 1\nLock Claimed"() -> (w249:refnum<vi>)
  n492 = control-ref of="Shared 2\nLock Claimed"() -> (w248:refnum<vi>)
  n493 = control-ref of="Pressure Limit Tripped 1"() -> (w374:refnum<vi>)
  n494 = control-ref of="Pressure Limit Tripped 2"() -> (w373:refnum<vi>)
  n495 = control-ref of="Pressure Limit Tripped 3"() -> (w372:refnum<vi>)
  n496 = control-ref of="Pressure Limit Tripped 4"() -> (w371:refnum<vi>)
  n497 = control-ref of="Pressure Limit Tripped 5"() -> (w370:refnum<vi>)
  n498 = control-ref of="Pressure Limit Tripped 6"() -> (w369:refnum<vi>)
  n499 = control-ref of="Recorded Pressure"() -> (w309:refnum<vi>)
  n500 = control-ref of="Recorded Pressure 2"() -> (w308:refnum<vi>)
  n501 = control-ref of="Recorded Pressure 3"() -> (w307:refnum<vi>)
  n502 = control-ref of="Recorded Pressure 4"() -> (w306:refnum<vi>)
  n503 = control-ref of="Recorded Pressure 5"() -> (w305:refnum<vi>)
  n504 = control-ref of="Recorded Pressure 6"() -> (w304:refnum<vi>)
  n505 = Build Array(w261, w259, w260, w258, w257, w256) -> (→"Last Cycle Temp Read Success Array":refnum<vi>[])
  n506 = control-ref of="Username 6"() -> (w204:refnum<vi>)
  n507 = control-ref of="Username 5"() -> (w203:refnum<vi>)
  n508 = control-ref of="Username 4"() -> (w202:refnum<vi>)
  n509 = control-ref of="Username 3"() -> (w201:refnum<vi>)
  n510 = control-ref of="Username 2"() -> (w200:refnum<vi>)
  n511 = control-ref of="Username 1"() -> (w199:refnum<vi>)
  n512 = Build Array(w250, w249, w248) -> (→"Pump Shared Lock\nClaimed Array":refnum<vi>[])
  n513 = control-ref of="Queue Reactor 6"() -> (w177:refnum<vi>)
  n514 = control-ref of="Queue Reactor 5"() -> (w176:refnum<vi>)
  n515 = control-ref of="Queue Reactor 4"() -> (w175:refnum<vi>)
  n516 = control-ref of="Queue Reactor 3"() -> (w174:refnum<vi>)
  n517 = control-ref of="Queue Reactor 2"() -> (w173:refnum<vi>)
  n518 = control-ref of="Queue Reactor 1"() -> (w172:refnum<vi>)
  n519 = control-ref of="Reactor 1 Errors"() -> (w330:refnum<vi>)
  n520 = control-ref of="Reactor 2 Errors"() -> (w329:refnum<vi>)
  n521 = control-ref of="Reactor 3 Errors"() -> (w328:refnum<vi>)
  n522 = control-ref of="Reactor 4 Errors"() -> (w327:refnum<vi>)
  n523 = control-ref of="Reactor 5 Errors"() -> (w326:refnum<vi>)
  n524 = control-ref of="Reactor 6 Errors"() -> (w325:refnum<vi>)
  n525 = Build Array(w309, w308, w307, w306, w305, w304) -> (→"Recorded Pressure Array":refnum<vi>[])
  n526 = Build Array(w374, w373, w372, w371, w370, w369) -> (→"Pressure Limit Tripped Array":refnum<vi>[])
  n527 = Build Array(w90, w85, w89, w88, w87, w86) -> (→"Local Connection JSON Array":refnum<vi>[])
  n528 = Build Array(w199, w200, w201, w202, w203, w204) -> (→"Username Array":refnum<vi>[])
  n529 = Build Array(w330, w329, w328, w327, w326, w325) -> (→"Reactor Errors Array":refnum<vi>[])
  n530 = control-ref of="Load Table Reactor 1"() -> (w161:refnum<vi>)
  n531 = control-ref of="Load Table Reactor 2"() -> (w160:refnum<vi>)
  n532 = control-ref of="Load Table Reactor 3"() -> (w159:refnum<vi>)
  n533 = control-ref of="Load Table Reactor 5"() -> (w122:refnum<vi>)
  n534 = control-ref of="Load Table Reactor 4"() -> (w121:refnum<vi>)
  n535 = control-ref of="Load Table Reactor 6"() -> (w158:refnum<vi>)
  n536 = control-ref of="Current Cycle 5"() -> (w398:refnum<vi>)
  n537 = control-ref of="Current Cycle 6"() -> (w397:refnum<vi>)
  n538 = control-ref of="Current Cycle 4"() -> (w399:refnum<vi>)
  n539 = control-ref of="Current Cycle 3"() -> (w400:refnum<vi>)
  n540 = control-ref of="Current Cycle 2"() -> (w401:refnum<vi>)
  n541 = control-ref of="Current Cycle 1"() -> (w402:refnum<vi>)
  n542 = Build Array(w172, w173, w174, w175, w176, w177) -> (→"Queue Array":refnum<vi>[])
  n543 = control-ref of="ALD Sequence for Reactor 1"() -> (w409:refnum<vi>)
  n544 = control-ref of="ALD Sequence for Reactor 2"() -> (w408:refnum<vi>)
  n545 = control-ref of="ALD Sequence for Reactor 3"() -> (w407:refnum<vi>)
  n546 = control-ref of="ALD Sequence for Reactor 4"() -> (w406:refnum<vi>)
  n547 = control-ref of="ALD Sequence for Reactor 5"() -> (w405:refnum<vi>)
  n548 = control-ref of="ALD Sequence for Reactor 6"() -> (w404:refnum<vi>)
  n549 = Build Array(w402, w401, w400, w399, w398, w397) -> (→"Current Cycle Display Array":refnum<vi>[])
  n550 = control-ref of="Time Elapsed (s) 1"() -> (w120:refnum<vi>)
  n551 = control-ref of="Time Elapsed (s) 2"() -> (w119:refnum<vi>)
  n552 = control-ref of="Time Elapsed (s) 3"() -> (w118:refnum<vi>)
  n553 = control-ref of="Time Elapsed (s) 4"() -> (w117:refnum<vi>)
  n554 = control-ref of="Time Elapsed (s) 5"() -> (w116:refnum<vi>)
  n555 = control-ref of="Time Elapsed (s) 6"() -> (w115:refnum<vi>)
  n556 = Build Array(w161, w160, w159, w121, w122, w158) -> (→"Load Table Reactor Array":refnum<vi>[])
  n557 = control-ref of="Manual Override\nPumps"() -> (w246:refnum<vi>)
  n558 = control-ref of="Manual Override\nShared1"() -> (w245:refnum<vi>)
  n559 = control-ref of="Manual Override\nShared2"() -> (w244:refnum<vi>)
  n560 = Build Array(w409, w408, w407, w406, w405, w404) -> (→"ALD Sequence for Reactor Array":refnum<vi>[])
  n561 = control-ref of="Pressure Tolerance Tripped 1"() -> (w367:refnum<vi>)
  n562 = control-ref of="Pressure Tolerance Tripped 2"() -> (w366:refnum<vi>)
  n563 = control-ref of="Pressure Tolerance Tripped 3"() -> (w365:refnum<vi>)
  n564 = control-ref of="Pressure Tolerance Tripped 4"() -> (w364:refnum<vi>)
  n565 = control-ref of="Pressure Tolerance Tripped 5"() -> (w363:refnum<vi>)
  n566 = control-ref of="Pressure Tolerance Tripped 6"() -> (w362:refnum<vi>)
  n567 = control-ref of="Logging Data 1"() -> (w337:refnum<vi>)
  n568 = control-ref of="Logging Data 2"() -> (w336:refnum<vi>)
  n569 = control-ref of="Logging Data 3"() -> (w335:refnum<vi>)
  n570 = control-ref of="Logging Data 4"() -> (w334:refnum<vi>)
  n571 = control-ref of="Logging Data 5"() -> (w333:refnum<vi>)
  n572 = control-ref of="Logging Data 6"() -> (w332:refnum<vi>)
  n573 = control-ref of="Error Trip Time"() -> (w282:refnum<vi>)
  n574 = control-ref of="Error Trip Time 2"() -> (w281:refnum<vi>)
  n575 = control-ref of="Error Trip Time 3"() -> (w280:refnum<vi>)
  n576 = control-ref of="Error Trip Time 4"() -> (w279:refnum<vi>)
  n577 = control-ref of="Error Trip Time 5"() -> (w278:refnum<vi>)
  n578 = control-ref of="Error Trip Time 6"() -> (w277:refnum<vi>)
  n579 = Build Array(w120, w119, w118, w117, w116, w115) -> (→"Time Elapsed Array":refnum<vi>[])
  n580 = Build Array(w246, w245, w244) -> (→"Manual Override\nPump Shared Array":refnum<vi>[])
  n581 = control-ref of="Pressure Graph 1"() -> (w323:refnum<vi>)
  n582 = control-ref of="Pressure Graph 2"() -> (w322:refnum<vi>)
  n583 = control-ref of="Pressure Graph 3"() -> (w321:refnum<vi>)
  n584 = control-ref of="Pressure Graph 4"() -> (w320:refnum<vi>)
  n585 = control-ref of="Pressure Graph 5"() -> (w319:refnum<vi>)
  n586 = control-ref of="Pressure Graph 6"() -> (w318:refnum<vi>)
  n587 = control-ref of="Timer Reactor 6"() -> (w163:refnum<vi>)
  n588 = control-ref of="Timer Reactor 5"() -> (w164:refnum<vi>)
  n589 = control-ref of="Timer Reactor 4"() -> (w165:refnum<vi>)
  n590 = control-ref of="Timer Reactor 3"() -> (w166:refnum<vi>)
  n591 = control-ref of="Timer Reactor 2"() -> (w167:refnum<vi>)
  n592 = control-ref of="Timer Reactor 1"() -> (w168:refnum<vi>)
  n593 = control-ref of="Local Connection txt 1"() -> (w97:refnum<vi>)
  n594 = control-ref of="Local Connection txt 2"() -> (w96:refnum<vi>)
  n595 = control-ref of="Local Connection txt 3"() -> (w95:refnum<vi>)
  n596 = control-ref of="Local Connection txt 4"() -> (w94:refnum<vi>)
  n597 = control-ref of="Local Connection txt 5"() -> (w93:refnum<vi>)
  n598 = control-ref of="Local Connection txt 6"() -> (w92:refnum<vi>)
  n599 = Build Array(w337, w336, w335, w334, w333, w332) -> (→"Logging Data Array":refnum<vi>[])
  n600 = Build Array(w323, w322, w321, w320, w319, w318) -> (→"Pressure Graph Array":refnum<vi>[])
  n601 = Build Array(w367, w366, w365, w364, w363, w362) -> (→"Pressure Tolerance Tripped Array":refnum<vi>[])
  n602 = Build Array(w168, w167, w166, w165, w164, w163) -> (→"Timer Reactor Array":refnum<vi>[])
  n603 = Build Array(w282, w281, w280, w279, w278, w277) -> (→"Error Trip Time\nArray":refnum<vi>[])
  n604 = control-ref of="Completion 5"() -> (w391:refnum<vi>)
  n605 = control-ref of="Completion 6"() -> (w390:refnum<vi>)
  n606 = control-ref of="Completion 4"() -> (w392:refnum<vi>)
  n607 = control-ref of="Completion 1"() -> (w395:refnum<vi>)
  n608 = control-ref of="Completion 2"() -> (w394:refnum<vi>)
  n609 = control-ref of="Completion 3"() -> (w393:refnum<vi>)
  n610 = Build Array(w97, w96, w95, w94, w93, w92) -> (→"Local Connection txt Array":refnum<vi>[])
  n611 = control-ref of="Save Table Reactor 6"() -> (w157:refnum<vi>)
  n612 = control-ref of="Save Table Reactor 5"() -> (w156:refnum<vi>)
  n613 = control-ref of="Save Table Reactor 4"() -> (w155:refnum<vi>)
  n614 = control-ref of="Save Table Reactor 3"() -> (w154:refnum<vi>)
  n615 = control-ref of="Save Table Reactor 2"() -> (w153:refnum<vi>)
  n616 = control-ref of="Save Table Reactor 1"() -> (w152:refnum<vi>)
  n617 = control-ref of="GUID 1"() -> (w104:refnum<vi>)
  n618 = control-ref of="GUID 2"() -> (w103:refnum<vi>)
  n619 = control-ref of="GUID 3"() -> (w102:refnum<vi>)
  n620 = control-ref of="GUID 4"() -> (w101:refnum<vi>)
  n621 = control-ref of="GUID 5"() -> (w100:refnum<vi>)
  n622 = control-ref of="GUID 6"() -> (w99:refnum<vi>)
  n623 = Build Array(w395, w394, w393, w392, w391, w390) -> (→"Completion Array":refnum<vi>[])
  n624 = Build Array(w104, w103, w102, w101, w100, w99) -> (→"GUID array":refnum<vi>[])
  n625 = control-ref of="Countdown 1"() -> (w213:refnum<vi>)
  n626 = control-ref of="Countdown 2"() -> (w214:refnum<vi>)
  n627 = control-ref of="Countdown 3"() -> (w218:refnum<vi>)
  n628 = control-ref of="Countdown 4"() -> (w217:refnum<vi>)
  n629 = control-ref of="Countdown 5"() -> (w216:refnum<vi>)
  n630 = control-ref of="Countdown 6"() -> (w215:refnum<vi>)
  n631 = control-ref of="Error Trip Cycle 3"() -> (w273:refnum<vi>)
  n632 = control-ref of="Error Trip Cycle 4"() -> (w272:refnum<vi>)
  n633 = control-ref of="Error Trip Cycle 1"() -> (w275:refnum<vi>)
  n634 = control-ref of="Error Trip Cycle 2"() -> (w274:refnum<vi>)
  n635 = control-ref of="Error Trip Cycle 6"() -> (w270:refnum<vi>)
  n636 = control-ref of="Error Trip Cycle 5"() -> (w271:refnum<vi>)
  n637 = control-ref of="System Idle 1"() -> (w344:refnum<vi>)
  n638 = control-ref of="System Idle 2"() -> (w343:refnum<vi>)
  n639 = control-ref of="System Idle 3"() -> (w342:refnum<vi>)
  n640 = control-ref of="System Idle 4"() -> (w341:refnum<vi>)
  n641 = control-ref of="System Idle 5"() -> (w340:refnum<vi>)
  n642 = control-ref of="System Idle 6"() -> (w339:refnum<vi>)
  n643 = control-ref of="Table Position Reactor 1"() -> (w360:refnum<vi>)
  n644 = control-ref of="Table Position Reactor 2"() -> (w359:refnum<vi>)
  n645 = control-ref of="Table Position Reactor 3"() -> (w358:refnum<vi>)
  n646 = control-ref of="Table Position Reactor 4"() -> (w357:refnum<vi>)
  n647 = control-ref of="Table Position Reactor 5"() -> (w356:refnum<vi>)
  n648 = control-ref of="Table Position Reactor 6"() -> (w355:refnum<vi>)
  n649 = Build Array(w152, w153, w154, w155, w156, w157) -> (→"Save Table Reactor Array":refnum<vi>[])
  n650 = Build Array(w213, w214, w218, w217, w216, w215) -> (→"Countdown Array":refnum<vi>[])
  n651 = control-ref of="Set Temperature 6"() -> (w291:refnum<vi>)
  n652 = control-ref of="Set Temperature 4"() -> (w293:refnum<vi>)
  n653 = control-ref of="Set Temperature 5"() -> (w292:refnum<vi>)
  n654 = control-ref of="Set Temperature 2"() -> (w295:refnum<vi>)
  n655 = control-ref of="Set Temperature 3"() -> (w294:refnum<vi>)
  n656 = control-ref of="Set Temperature"() -> (w296:refnum<vi>)
  n657 = control-ref of="Temperature Graph 1"() -> (w316:refnum<vi>)
  n658 = control-ref of="Temperature Graph 2"() -> (w315:refnum<vi>)
  n659 = control-ref of="Temperature Graph 3"() -> (w314:refnum<vi>)
  n660 = control-ref of="Temperature Graph 4"() -> (w313:refnum<vi>)
  n661 = control-ref of="Temperature Graph 5"() -> (w312:refnum<vi>)
  n662 = control-ref of="Temperature Graph 6"() -> (w311:refnum<vi>)
  n663 = Build Array(w275, w274, w273, w272, w271, w270) -> (→"Error Trip Cycle\nArray":refnum<vi>[])
  n664 = Build Array(w344, w343, w342, w341, w340, w339) -> (→"System Idle Array":refnum<vi>[])
  n665 = Build Array(w360, w359, w358, w357, w356, w355) -> (→"Table Position Reactor Array":refnum<vi>[])
  n666 = control-ref of="Temp Setpoint"() -> (w289:refnum<vi>)
  n667 = control-ref of="Temp Setpoint 2"() -> (w288:refnum<vi>)
  n668 = control-ref of="Temp Setpoint 3"() -> (w287:refnum<vi>)
  n669 = control-ref of="Temp Setpoint 4"() -> (w286:refnum<vi>)
  n670 = control-ref of="Temp Setpoint 5"() -> (w285:refnum<vi>)
  n671 = control-ref of="Temp Setpoint 6"() -> (w284:refnum<vi>)
  n672 = control-ref of="Last Temperature\nRead Success Time 6"() -> (w263:refnum<vi>)
  n673 = control-ref of="Last Temperature\nRead Success Time 5"() -> (w264:refnum<vi>)
  n674 = control-ref of="Last Temperature\nRead Success Time 4"() -> (w265:refnum<vi>)
  n675 = control-ref of="Last Temperature\nRead Success Time 3"() -> (w266:refnum<vi>)
  n676 = control-ref of="Last Temperature\nRead Success Time 2"() -> (w267:refnum<vi>)
  n677 = Build Array(w296, w295, w294, w293, w292, w291) -> (→"Set Temperature Array":refnum<vi>[])
  n678 = control-ref of="Last Temperature\nRead Success Time"() -> (w268:refnum<vi>)
  n679 = Build Array(w316, w315, w314, w313, w312, w311) -> (→"Temperature Graph Array":refnum<vi>[])
  n680 = Build Array(w289, w288, w287, w286, w285, w284) -> (→"Temp Setpoint Array":refnum<vi>[])
  n681 = Build Array(w268, w267, w266, w265, w264, w263) -> (→"Last Temperature\nReat Success Time\nArray":refnum<vi>[])
  n682 = control-ref of="Time Left 6"() -> (w383:refnum<vi>)
  n683 = control-ref of="Time Left 5"() -> (w384:refnum<vi>)
  n684 = control-ref of="Time Left 4"() -> (w385:refnum<vi>)
  n685 = control-ref of="Time Left 3"() -> (w386:refnum<vi>)
  n686 = control-ref of="Time Left 1"() -> (w388:refnum<vi>)
  n687 = control-ref of="Time Left 2"() -> (w387:refnum<vi>)
  n688 = control-ref of="Stop / Start Reactor 1"() -> (w416:refnum<vi>)
  n689 = control-ref of="Stop / Start Reactor 2"() -> (w415:refnum<vi>)
  n690 = control-ref of="Stop / Start Reactor 3"() -> (w414:refnum<vi>)
  n691 = control-ref of="Stop / Start Reactor 4"() -> (w413:refnum<vi>)
  n692 = control-ref of="Stop / Start Reactor 5"() -> (w412:refnum<vi>)
  n693 = control-ref of="Stop / Start Reactor 6"() -> (w411:refnum<vi>)
  n694 = control-ref of="Experimental Details 6"() -> (w151:refnum<vi>)
  n695 = control-ref of="Experimental Details 1"() -> (w150:refnum<vi>)
  n696 = control-ref of="Experimental Details 5"() -> (w149:refnum<vi>)
  n697 = control-ref of="Experimental Details 4"() -> (w148:refnum<vi>)
  n698 = control-ref of="Experimental Details 3"() -> (w147:refnum<vi>)
  n699 = control-ref of="Experimental Details 2"() -> (w146:refnum<vi>)
  n700 = Build Array(w388, w387, w386, w385, w384, w383) -> (→"Time Left Array":refnum<vi>[])
  n701 = Build Array(w416, w415, w414, w413, w412, w411) -> (→"Start Stop Reactor Array":refnum<vi>[])
  n702 = control-ref of="Start Time 6"() -> (w145:refnum<vi>)
  n703 = control-ref of="Start Time 5"() -> (w144:refnum<vi>)
  n704 = control-ref of="Start Time 4"() -> (w143:refnum<vi>)
  n705 = control-ref of="Start Time 3"() -> (w142:refnum<vi>)
  n706 = control-ref of="Start Time 2"() -> (w141:refnum<vi>)
  n707 = control-ref of="Start Time 1"() -> (w140:refnum<vi>)
  n708 = control-ref of="Pressure (mTorr) 1"() -> (w302:refnum<vi>)
  n709 = control-ref of="Pressure (mTorr) 2"() -> (w301:refnum<vi>)
  n710 = control-ref of="Pressure (mTorr) 3"() -> (w300:refnum<vi>)
  n711 = control-ref of="Pressure (mTorr) 4"() -> (w299:refnum<vi>)
  n712 = control-ref of="Pressure (mTorr) 5"() -> (w298:refnum<vi>)
  n713 = control-ref of="Pressure (mTorr) 6"() -> (w297:refnum<vi>)
  n714 = Build Array(w150, w146, w147, w148, w149, w151) -> (→"Experimental Details Array":refnum<vi>[])
  n715 = control-ref of="Current Cycle Reactor 6"() -> (w350:refnum<vi>)
  n716 = control-ref of="Current Cycle Reactor 5"() -> (w349:refnum<vi>)
  n717 = control-ref of="Current Cycle Reactor 3"() -> (w351:refnum<vi>)
  n718 = control-ref of="Current Cycle Reactor 4"() -> (w348:refnum<vi>)
  n719 = control-ref of="Current Cycle Reactor 2"() -> (w352:refnum<vi>)
  n720 = control-ref of="Current Cycle Reactor 1"() -> (w353:refnum<vi>)
  n721 = control-ref of="Save File Connection 4"() -> (w206:refnum<vi>)
  n722 = control-ref of="Save File Connection 5"() -> (w207:refnum<vi>)
  n723 = control-ref of="Save File Connection 6"() -> (w208:refnum<vi>)
  n724 = control-ref of="Save File Connection 3"() -> (w209:refnum<vi>)
  n725 = control-ref of="Save File Connection 2"() -> (w210:refnum<vi>)
  n726 = control-ref of="Save File Connection 1"() -> (w211:refnum<vi>)
  n727 = control-ref of="Save File JSON Connection 4"() -> (w126:refnum<vi>)
  n728 = control-ref of="Save File JSON Connection 5"() -> (w125:refnum<vi>)
  n729 = control-ref of="Save File JSON Connection 6"() -> (w124:refnum<vi>)
  n730 = control-ref of="Save File JSON Connection 3"() -> (w127:refnum<vi>)
  n731 = control-ref of="Save File JSON Connection 2"() -> (w128:refnum<vi>)
  n732 = control-ref of="Save File JSON Connection 1"() -> (w129:refnum<vi>)
  n733 = Build Array(w140, w141, w142, w143, w144, w145) -> (→"Start Time Array":refnum<vi>[])
  n734 = Build Array(w302, w301, w300, w299, w298, w297) -> (→"Pressure (mTorr) Array":refnum<vi>[])
  n735 = Build Array(w211, w210, w209, w206, w207, w208) -> (→"Save File Connection Array":refnum<vi>[])
  n736 = control-ref of="Chamber 1 Lock Claimed"() -> (w252:refnum<vi>)
  n737 = control-ref of="Chamber 2 Lock Claimed"() -> (w237:refnum<vi>)
  n738 = control-ref of="Chamber 3 Lock Claimed"() -> (w236:refnum<vi>)
  n739 = control-ref of="Chamber 4 Lock Claimed"() -> (w235:refnum<vi>)
  n740 = control-ref of="Chamber 5 Lock Claimed"() -> (w234:refnum<vi>)
  n741 = control-ref of="Chamber 6 Lock Claimed"() -> (w233:refnum<vi>)
  n742 = Build Array(w353, w352, w351, w348, w349, w350) -> (→"Current Cycle Reactor Array":refnum<vi>[])
  n743 = control-ref of="Manual Override Chamber 1"() -> (w254:refnum<vi>)
  n744 = control-ref of="Manual Override Chamber 2"() -> (w242:refnum<vi>)
  n745 = control-ref of="Manual Override Chamber 3"() -> (w241:refnum<vi>)
  n746 = control-ref of="Manual Override Chamber 4"() -> (w240:refnum<vi>)
  n747 = control-ref of="Manual Override Chamber 5"() -> (w239:refnum<vi>)
  n748 = control-ref of="Manual Override Chamber 6"() -> (w238:refnum<vi>)
  n749 = control-ref of="Wait Before Start (s) 1"() -> (w381:refnum<vi>)
  n750 = control-ref of="Wait Before Start (s) 2"() -> (w380:refnum<vi>)
  n751 = control-ref of="Wait Before Start (s) 3"() -> (w379:refnum<vi>)
  n752 = control-ref of="Wait Before Start (s) 4"() -> (w378:refnum<vi>)
  n753 = control-ref of="Wait Before Start (s) 5"() -> (w377:refnum<vi>)
  n754 = control-ref of="Wait Before Start (s) 6"() -> (w376:refnum<vi>)
  n755 = Build Array(w129, w128, w127, w126, w125, w124) -> (→"Save File JSON Connection Array":refnum<vi>[])
  n756 = local write "Stop / Start Reactor 6"(w196) -> ()
  n757 = local write "Stop / Start Reactor 5"(w196) -> ()
  n758 = local write "Stop / Start Reactor 4"(w196) -> ()
  n759 = local write "Stop / Start Reactor 3"(w196) -> ()
  n760 = local write "Stop / Start Reactor 2"(w196) -> ()
  n761 = local write "Stop / Start Reactor 1"(w196) -> ()
  n762 = Build Array(w252, w237, w236, w235, w234, w233) -> (→"Chamber Lock Claimed Array":refnum<vi>[])
  n763 = Build Array(w381, w380, w379, w378, w377, w376) -> (→"Wait Before Start Array":refnum<vi>[])
  n764 = Build Array(w254, w242, w241, w240, w239, w238) -> (→"Manual Override\nChamber Array":refnum<vi>[])
  n765 = control-ref of="Running Reactor 1"() -> (w17:refnum<vi>)
  n766 = control-ref of="Running Reactor 6"() -> (w12:refnum<vi>)
  n767 = control-ref of="Running Reactor 5"() -> (w13:refnum<vi>)
  n768 = control-ref of="Running Reactor 4"() -> (w14:refnum<vi>)
  n769 = control-ref of="Running Reactor 3"() -> (w15:refnum<vi>)
  n770 = control-ref of="Running Reactor 2"() -> (w16:refnum<vi>)
  n771 = Build Array(w17, w16, w15, w14, w13, w12) -> (→"Running Reactor\nIndicator Array":refnum<vi>[])
  n772 = control-ref of="Pressure Voltage Correct 1"() -> (w73:refnum<vi>)
  n773 = control-ref of="Pressure Voltage Correct 2"() -> (w74:refnum<vi>)
  n774 = control-ref of="Pressure Voltage Correct 3"() -> (w75:refnum<vi>)
  n775 = control-ref of="Pressure Voltage Correct 4"() -> (w76:refnum<vi>)
  n776 = control-ref of="Pressure Voltage Correct 5"() -> (w77:refnum<vi>)
  n777 = control-ref of="Pressure Voltage Correct 6"() -> (w78:refnum<vi>)
  n778 = control-ref of="Pressure Scale 1"() -> (w72:refnum<vi>)
  n779 = control-ref of="Pressure Scale 2"() -> (w71:refnum<vi>)
  n780 = control-ref of="Pressure Scale 3"() -> (w70:refnum<vi>)
  n781 = control-ref of="Pressure Scale 4"() -> (w69:refnum<vi>)
  n782 = control-ref of="Pressure Scale 5"() -> (w68:refnum<vi>)
  n783 = control-ref of="Pressure Scale 6"() -> (w67:refnum<vi>)
  n784 = Build Array(w73, w74, w75, w76, w77, w78) -> (→"Pressure Voltage\nCorrect Array":refnum<vi>[])
  n785 = Build Array(w72, w71, w70, w69, w68, w67) -> (→"Pressure Scale Array":refnum<vi>[])
  n786 = control-ref of="Manual 44"() -> (w132:refnum<vi>)
  n787 = control-ref of="Manual 43"() -> (w133:refnum<vi>)
  n788 = control-ref of="Manual 42"() -> (w134:refnum<vi>)
  n789 = control-ref of="Manual 41"() -> (w135:refnum<vi>)
  n790 = control-ref of="Manual 40"() -> (w136:refnum<vi>)
  n791 = control-ref of="Manual 39"() -> (w137:refnum<vi>)
  n792 = control-ref of="Manual 38"() -> (w138:refnum<vi>)
  n793 = control-ref of="Manual 37"() -> (w139:refnum<vi>)
  n794 = control-ref of="Manual 45"() -> (w10:refnum<vi>)
  n795 = control-ref of="Manual 46"() -> (w9:refnum<vi>)
  n796 = control-ref of="Manual 47"() -> (w4:refnum<vi>)
  n797 = control-ref of="Manual 48"() -> (w3:refnum<vi>)
  n798 = control-ref of="Header Connection txt 1"() -> (w113:refnum<vi>)
  n799 = control-ref of="Header Connection txt 2"() -> (w112:refnum<vi>)
  n800 = control-ref of="Header Connection txt 3"() -> (w111:refnum<vi>)
  n801 = control-ref of="Header Connection txt 4"() -> (w110:refnum<vi>)
  n802 = control-ref of="Header Connection txt 5"() -> (w109:refnum<vi>)
  n803 = control-ref of="Header Connection txt 6"() -> (w108:refnum<vi>)
  n804 = Build Array(w139, w138, w137, w136, w135, w134, w133, w132, w10, w9, w4, w3) -> (→"Shared Manual Valve Array":refnum<vi>[])
  n805 = Build Array(w113, w112, w111, w110, w109, w108) -> (→"Header Connection txt Array":refnum<vi>[])
  n806 = control-ref of="Valve 14"() -> (w49:refnum<vi>)
  n807 = control-ref of="Valve 13"() -> (w50:refnum<vi>)
  n808 = control-ref of="Valve 12"() -> (w51:refnum<vi>)
  n809 = control-ref of="Valve 11"() -> (w52:refnum<vi>)
  n810 = control-ref of="Valve 10"() -> (w53:refnum<vi>)
  n811 = control-ref of="Valve 9"() -> (w54:refnum<vi>)
  n812 = control-ref of="Valve 8"() -> (w55:refnum<vi>)
  n813 = control-ref of="Valve 7"() -> (w56:refnum<vi>)
  n814 = control-ref of="Valve 6"() -> (w57:refnum<vi>)
  n815 = control-ref of="Valve 5"() -> (w58:refnum<vi>)
  n816 = control-ref of="Valve 4"() -> (w59:refnum<vi>)
  n817 = control-ref of="Valve 3"() -> (w60:refnum<vi>)
  n818 = control-ref of="Valve 2"() -> (w61:refnum<vi>)
  n819 = control-ref of="Valve 1"() -> (w62:refnum<vi>)
  n820 = control-ref of="Valve 28"() -> (w35:refnum<vi>)
  n821 = control-ref of="Valve 27"() -> (w36:refnum<vi>)
  n822 = control-ref of="Valve 26"() -> (w37:refnum<vi>)
  n823 = control-ref of="Valve 25"() -> (w38:refnum<vi>)
  n824 = control-ref of="Valve 24"() -> (w39:refnum<vi>)
  n825 = control-ref of="Valve 23"() -> (w40:refnum<vi>)
  n826 = control-ref of="Valve 22"() -> (w41:refnum<vi>)
  n827 = control-ref of="Valve 21"() -> (w42:refnum<vi>)
  n828 = control-ref of="Valve 20"() -> (w43:refnum<vi>)
  n829 = control-ref of="Valve 19"() -> (w44:refnum<vi>)
  n830 = control-ref of="Valve 18"() -> (w45:refnum<vi>)
  n831 = control-ref of="Valve 17"() -> (w46:refnum<vi>)
  n832 = control-ref of="Valve 16"() -> (w47:refnum<vi>)
  n833 = control-ref of="Valve 15"() -> (w48:refnum<vi>)
  n834 = control-ref of="Valve 42"() -> (w21:refnum<vi>)
  n835 = control-ref of="Valve 41"() -> (w22:refnum<vi>)
  n836 = control-ref of="Valve 40"() -> (w23:refnum<vi>)
  n837 = control-ref of="Valve 39"() -> (w24:refnum<vi>)
  n838 = control-ref of="Valve 38"() -> (w25:refnum<vi>)
  n839 = control-ref of="Valve 37"() -> (w26:refnum<vi>)
  n840 = control-ref of="Valve 36"() -> (w27:refnum<vi>)
  n841 = control-ref of="Valve 35"() -> (w28:refnum<vi>)
  n842 = control-ref of="Valve 34"() -> (w29:refnum<vi>)
  n843 = control-ref of="Valve 33"() -> (w30:refnum<vi>)
  n844 = control-ref of="Valve 32"() -> (w31:refnum<vi>)
  n845 = control-ref of="Valve 31"() -> (w32:refnum<vi>)
  n846 = control-ref of="Valve 30"() -> (w33:refnum<vi>)
  n847 = control-ref of="Valve 29"() -> (w34:refnum<vi>)
  n848 = control-ref of="Valve 47"() -> (w6:refnum<vi>)
  n849 = control-ref of="Valve 48"() -> (w5:refnum<vi>)
  n850 = control-ref of="Valve 46"() -> (w7:refnum<vi>)
  n851 = control-ref of="Valve 45"() -> (w8:refnum<vi>)
  n852 = control-ref of="Valve 44"() -> (w20:refnum<vi>)
  n853 = control-ref of="Valve 43"() -> (w18:refnum<vi>)
  n854 = Build Array(w62, w61, w60, w59, w58, w57, w56, w55, w54, w53, w52, w51, w50, w49, w48, w47, w46, w45, w44, w43, w42, w41, w40, w39, w38, w37, w36, w35, w34, w33, w32, w31, w30, w29, w28, w27, w26, w25, w24, w23, w22, w21, w18, w20, w8, w7, w6, w5) -> (→"Valve Indicator Array":refnum<vi>[])
  n855 = disable-structure shown="Disabled" {
    frame Disabled {
      # "code that writes a log message for any changes made in the experiemtnal details table"
      # "check if the table changes and if it does then add to message log"
      n856 = local read "Number of Reactors"() -> (w1115:i32)
      n857 = control-ref of="ALD Sequence for Reactor Array"() -> (w1116:refnum<vi>)
      n858 = control-ref of="GUID array"() -> (w1113:refnum<vi>)
      n859 = control-ref of="Logging Data Array"() -> (w1109:refnum<vi>)
      n860 = control-ref of="Queue Array"() -> (w1111:refnum<vi>)
      n861 = property class="Arr (strict)"(reference=w1111) -> ("Value"=w1110:refnum<vi>[])  [unwired: 1 in, 2 out]
      n862 = property class="Arr (strict)"(reference=w1116) -> ("Value"=w1114:refnum<vi>[])  [unwired: 1 in, 2 out]
      n863 = property class="Arr (strict)"(reference=w1113) -> ("Value"=w1112:refnum<vi>[])  [unwired: 1 in, 2 out]
      n864 = property class="Arr (strict)"(reference=w1109) -> ("Value"=w1108:refnum<vi>[])  [unwired: 1 in, 2 out]
      n865 = for {
        N: w1115 -> [_]
        workers-P: w1115 -> [_]
        tunnel: w1114 -> [w1120] mode=indexing
        tunnel: w1112 -> [w1119] mode=indexing
        tunnel: w1110 -> [w1118] mode=indexing
        tunnel: w1108 -> [w1117] mode=indexing
        n866 = while {
          tunnel: w1120 -> [w1127]
          tunnel: w1119 -> [w1125]
          tunnel: w1118 -> [w1124]
          tunnel: w1117 -> [w1123]
          stop <- FALSE stop-if-true
          n867 = property class="Bool (strict)"(reference=w1123) -> ("Value"=w1122:bool)  [unwired: 1 in, 2 out]
          n868 = Wait (ms)(milliseconds to wait=u32 100) -> ()  [unwired: 1 out]
          n869 = case shown="True" w1122 {
            tunnel: w1127 -> [_ w1133]
            tunnel: w1125 -> [_ w1130]
            tunnel: w1124 -> [_ w1128]
            frame False {
            }
            frame True {
              n870 = property class="Tbl (strict)"(reference=w1133) -> ("Value"=w1131:string[][])  [unwired: 1 in, 2 out]
              n871 = Decimal String To Number(string=w1131) -> (number=w1129:i32[][])  [unwired: 2 in, 1 out]
              n872 = call "Is Value Changed.vim"("value"=w1129) -> ("changed or first call?"=w1132:bool)
              n873 = case shown="True" w1132 {
                tunnel: w1130 -> [_ w1144]
                tunnel: w1129 -> [_ w1142]
                tunnel: w1128 -> [_ w1136]
                frame False {
                  # "table not changed do nothing"
                }
                frame True {
                  # "changed so add to log"
                  n874 = property class="Str"(reference=w1144) -> ("Value"=w1143:string)  [unwired: 1 in, 2 out]
                  n875 = Bundle By Name(cluster=cluster{"GUID":string, "valveSequence":i32[][]} {"GUID"="", "valveSequence"=[]} ("input cluster"), "GUID"=w1143, "valveSequence"=w1142) -> (w1140:cluster{"GUID":string, "valveSequence":i32[][]})
                  n876 = Bundle By Name(cluster=T7 {"type"="", "meta"="", "payload"={"GUID"="", "valveSequence"=[]}} ("input cluster"), "type"="recipe change", "payload"=w1140, "meta"="") -> (w1134:T7)
                  n877 = Flatten To JSON(anything=w1134) -> (JSON string=w1135:string)  [unwired: 2 in, 1 out]
                  n878 = property class="TypRef (strict)"(reference=w1136) -> ("Value"=w1139:refnum<queue>)  [unwired: 1 in, 2 out]
                  n879 = Enqueue Element(queue=w1139, element=w1135) -> ()  [unwired: 2 in, 3 out]
                }
              }
            }
          }
        }
      }
    }
    frame Enabled {
    }
  }
  n880 = disable-structure shown="Disabled" {
    frame Disabled {
      # "Consumer loop for the JSON objects"
      n881 = while {
        stop <- FALSE stop-if-true
        n882 = control-ref of="Save JSON log Connection"() -> (w1146:refnum<vi>)
        n883 = control-ref of="Queue JSON Object"() -> (w1150:refnum<vi>)
        n884 = property class="Ref (strict)"(reference=w1146) -> ("Value"=w1147:refnum<file>)  [unwired: 1 in, 2 out]
        n885 = property class="TypRef (strict)"(reference=w1150) -> ("Value"=w1152:refnum<queue>)  [unwired: 1 in, 2 out]
        n886 = Dequeue Element(queue=w1152) -> (element=w1148:string, error out=w1149:errorcluster)  [unwired: 2 in, 2 out]
        n887 = case shown="No Error" w1149 {
          tunnel: w1148 -> [w1155 _]
          tunnel: w1147 -> [w1158 _]
          frame No Error {
            # "add new line"
            # "there is something in the queue"
            n888 = Set File Position(refnum=w1158, from (0:start)=enum16{"start", "end", "current"}."end") -> (refnum out=w1156:refnum<file>)  [unwired: 2 in, 1 out]
            n889 = Concatenate Strings(w1155, "\r") -> (w1154:string)
            n890 = Write to Text File(file (use dialog)=w1156, text=w1154) -> ()  [unwired: 2 in, 3 out]
          }
          frame Error {
          }
        }
      }
    }
    frame Enabled {
    }
  }
  n891 = disable-structure shown="Disabled" {
    frame Disabled {
      n892 = while {
        stop <- TRUE continue-if-true
        n893 = stacked-sequence {
          frame #0 {
            n894 = case shown="True" "Plot Temp" {
              frame False {
                n895 = Wait Until Next ms Multiple(millisecond multiple=u32 100) -> ()  [unwired: 1 out]
              }
              frame True {
                n896 = call "ReadControllerTemperature.vi"("VISA resource name"=refnum<visa-resource-name> "COM4") -> ("error out"=w1166:errorcluster, "Success?"=w1164:bool, "Temp"=w1163:dbl)  [unwired: 8 in]
                n897 = local write "Tempurature Error"(w1166) -> ()
                n898 = local write "Temperature Graph 1"(w1163) -> ()
                n899 = case shown="True" w1164 {
                  frame False {
                  }
                  frame True {
                    n900 = local read "Current Cycle Reactor 1"() -> (w1167:i32)
                    n901 = Get Date/Time In Seconds() -> (seconds since 1Jan1904=w1173:timestamp)
                    n902 = Get Date/Time String(date format (0)=enum16{"short", "long", "abbreviated"}."abbreviated", seconds (now)=w1173, want seconds? (F)=TRUE) -> (date string=w1169:string, time string=w1170:string)
                    n903 = Concatenate Strings(w1169, w1170) -> (w1168:string)
                    n904 = local write "Last Temperature\nRead Success Time"(w1168) -> ()
                    n905 = local write "Last Cycle Temp\nRead Success"(w1167) -> ()
                  }
                }
              }
            }
          }
          frame #1 {
            n906 = local read "Set Temperature"() -> (w1174:bool)
            n907 = case shown="True" w1174 {
              frame False {
              }
              frame True {
                n908 = local read "Temp Setpoint"() -> (w1175:dbl)
                n909 = call "SetControllerTemperature.vi"("Temp Setpoint"=w1175) -> ("error out"=→"Tempurature Error":errorcluster, "Success?"=w1176:bool)  [unwired: 9 in]
                n910 = case shown="True" w1176 {
                  frame False {
                  }
                  frame True {
                    n911 = local write "Set Temperature"(FALSE ("Set Tempreature")) -> ()
                  }
                }
              }
            }
          }
        }
        n912 = Wait Until Next ms Multiple(millisecond multiple=u32 100) -> ()  [unwired: 1 out]
      }
    }
    frame Enabled {
    }
  }
  n913 = disable-structure shown="Disabled" {
    disable-tunnel: [w1186 _] -> _
    disable-tunnel: [w1186 _] -> _
    frame Disabled {
      w1186 = path "g:/Shared drives/Bergsman Group Files/Data/Reactor Data" ("file path (use dialog)")
      n914 = Build Path() -> (appended path=w1183:path)  [unwired: 2 in]
      n915 = Build Path(name or relative path="JSON Files") -> (appended path=w1180:path)  [unwired: 1 in]
      n916 = call <vilib>:"Check if File or Folder Exists.vi"("path"=w1183) -> ("error out"=w1185:errorcluster, "dup path"=w1184:path)  [unwired: 8 in, 1 out]
      n917 = call <vilib>:"Check if File or Folder Exists.vi"("path"=w1180) -> ("error out"=w1182:errorcluster, "dup path"=w1181:path)  [unwired: 8 in, 1 out]
      n918 = Create Folder(path (use dialog)=w1184, error in=w1185) -> ()  [unwired: 1 in, 3 out]
      n919 = Create Folder(path (use dialog)=w1181, error in=w1182) -> ()  [unwired: 1 in, 3 out]
    }
    frame Enabled {
    }
  }
  "Countdown 1" <- 0.0 ("Countdown")
  "Reactor 1 Errors" <- w185
  "Time Left 2" <- w189
  "Completion 2" <- w190
  "Current Cycle 2" <- w191
  "Time Left 3" <- w189
  "Completion 3" <- w190
  "Current Cycle 3" <- w191
  "Current Cycle 1" <- w191
  "Completion 1" <- w190
  "Time Left 1" <- w189
  "Time Left 4" <- w189
  "Completion 4" <- w190
  "Current Cycle 4" <- w191
  "Time Left 5" <- w189
  "Completion 5" <- w190
  "Current Cycle 5" <- w191
  "Time Left 6" <- w189
  "Completion 6" <- w190
  "Current Cycle 6" <- w191
  "Pressure\nLimit\nTripped 1" <- w187
  "Pressure\nTolerance\nTripped 1" <- w186
  "Pressure\nTolerance\nTripped 2" <- w186
  "Pressure\nLimit\nTripped 2" <- w187
  "Pressure\nTolerance\nTripped 3" <- w186
  "Pressure\nLimit\nTripped 3" <- w187
  "Pressure\nTolerance\nTripped 4" <- w186
  "Pressure\nLimit\nTripped 4" <- w187
  "Pressure\nTolerance\nTripped 5" <- w186
  "Pressure\nLimit\nTripped 5" <- w187
  "Pressure\nTolerance\nTripped 6" <- w186
  "Pressure\nLimit\nTripped 6" <- w187
  "Current Cycle Reactor 1" <- w193
  "Table Position Reactor 1" <- w192
  "Table Position Reactor 2" <- w192
  "Table Position Reactor 3" <- w192
  "Table Position Reactor 4" <- w192
  "Table Position Reactor 5" <- w192
  "Table Position Reactor 6" <- w192
  "Current Cycle Reactor 2" <- w193
  "Current Cycle Reactor 3" <- w193
  "Current Cycle Reactor 4" <- w193
  "Current Cycle Reactor 5" <- w193
  "Current Cycle Reactor 6" <- w193
  "System Idle 1" <- w195
  "Logging Data 1" <- w194
  "Logging Data 2" <- w194
  "System Idle 2" <- w195
  "Logging Data 3" <- w194
  "System Idle 3" <- w195
  "Logging Data 4" <- w194
  "System Idle 4" <- w195
  "Logging Data 5" <- w194
  "System Idle 5" <- w195
  "Logging Data 6" <- w194
  "System Idle 6" <- w195
  "Reactor 2 Errors" <- w185
  "Reactor 3 Errors" <- w185
  "Reactor 4 Errors" <- w185
  "Reactor 5 Errors" <- w185
  "Reactor 6 Errors" <- w185
  "Pump\nLock Claimed" <- FALSE ("Pump\nLock Claimed")
  "Chamber 1 Lock Claimed" <- FALSE ("Chamber 1 Lock Claimed")
  "Shared 2\nLock Claimed" <- FALSE ("Shared 2\nLock Claimed")
  "Shared 1\nLock Claimed" <- FALSE ("Shared 1\nLock Claimed")
  "Chamber 2 Lock Claimed" <- FALSE ("Chamber 2 Lock Claimed")
  "Chamber 3 Lock Claimed" <- FALSE ("Chamber 3 Lock Claimed")
  "Chamber 4 Lock Claimed" <- FALSE ("Chamber 4 Lock Claimed")
  "Chamber 5 Lock Claimed" <- FALSE ("Chamber 5 Lock Claimed")
  "Chamber 6 Lock Claimed" <- FALSE ("Chamber 6 Lock Claimed")
  "Countdown 2" <- 0.0 ("Countdown")
  "Countdown 3" <- 0.0 ("Countdown")
  "Countdown 4" <- 0.0 ("Countdown")
  "Countdown 5" <- 0.0 ("Countdown")
  "Countdown 6" <- 0.0 ("Countdown")
  "Save File Connection 1" <- w188
  "Save File Connection 2" <- w188
  "Save File Connection 3" <- w188
  "Save File Connection 6" <- w188
  "Save File Connection 5" <- w188
  "Save File Connection 4" <- w188
  "System Log" <- string[] ["", "", "", "", "", "", "", "", "", "", "", "", "", "", "", "", "", "", "", "", " ", "", "", "", "", "", "", "", "", "", " "] ("System Log")
  "Timer Reactor 1" <- w169
  "Timer Reactor 2" <- w169
  "Timer Reactor 3" <- w169
  "Timer Reactor 4" <- w169
  "Timer Reactor 5" <- w169
  "Timer Reactor 6" <- w169
  "Start Time 1" <- w2
  "Start Time 2" <- w2
  "Start Time 3" <- w2
  "Start Time 4" <- w2
  "Start Time 5" <- w2
  "Start Time 6" <- w2
  "Save File JSON Connection 1" <- w105
  "Save File JSON Connection 2" <- w105
  "Save File JSON Connection 3" <- w105
  "Save File JSON Connection 6" <- w105
  "Save File JSON Connection 5" <- w105
  "Save File JSON Connection 4" <- w105
  "Header Connection txt 1" <- w107
  "Header Connection txt 2" <- w107
  "Header Connection txt 3" <- w107
  "Header Connection txt 4" <- w107
  "Header Connection txt 5" <- w107
  "Header Connection txt 6" <- w107
  "Save JSON log Connection" <- refnum<file> refnum ("Save File Connection 6")
